vi "AlliGator Load IRFs & Fit Data (Map) HDF5 File v0.7.vi"(8 "Error In":errorcluster, 9 "File Type & Version only":bool, 11 "File Path":path) -> (0 "error out":errorcluster, 1 "Data Description":string, 2 "Decay Fit Options & Parameters":T1={"SYNC Period"=0.0, "Fit Options"={"Show Fit Residuals"=FALSE, "Fit Model"=enum."1-Exponential", "Residual Type"=enum."Standard", "Max Decay Percentile"=0.0, "Min Decay Percentile"=0.0, "Show Full Decay"=FALSE, "Weights"=enum."Unweighted", "Fitting Method"=enum."Least Square", "Compute Parameter Uncertainties"=FALSE, "Periodic Boundaries"=FALSE, "Model Calculation"=enum."Simulation", "Period"=0.0, "Termination Criteria"={"Max Iterations"=0, "Max Function Calls"=0, "Max Time"=0.0, "Function Tolerance"=0.0, "Parameter Tolerance"=0.0, "Gradient Tolerance"=0.0, "Min Lambda"=0.0, "Max Lambda"=0.0, "Initial Tick Count"=0}, "Offset Resolution"=0.0, "Use Local IRF"=FALSE, "Fitting Algorithm"=enum."Levenberg-Marquardt", "Show Confidence Interval "=TRUE, "Confidence Level"=95.0}, "Fit Parameter Constraints"=[], "MLE Baseline Offset"=0.0, "MLE Baseline Offset Type"=enum."Absolute"} {"Fit Options"."Confidence Level" min=0.0 max=100.0; "Fit Options"."Offset Resolution" min=0.0; "Fit Options"."Period" min=0.0; "Fit Options"."Min Decay Percentile" min=0.0 max=1.0; "Fit Options"."Max Decay Percentile" min=0.0 max=100.0; "Fit Parameter Constraints"."Max Value" format="%#.3g"; "Fit Parameter Constraints"."Min Value" format="%#.3g"}, 3 "IRFs & Fit Data Map v3":T13 {"Fit Options: Decay Preprocessing Parameters"."# Folds" min=1}, 4 "[Multiple Decays Fit Parameters SDV]":dbl[][](array[numeric]), 5 "File Version":string, 7 "File Type":string)   [LabVIEW 2021, in "AlliGator Decay Fit Parameter Map.lvlib"]
doc: "Loads Decay Fit Parameter Map and associated metadata."
uses:
  AlliGator Decay Fit Parameter Map.lvlib
  AlliGator IRFs & Fit Data v3.ctl
  Fits/IRF(X)PSED/Decay Fit Parameters & Derived Quantities List v2.ctl
  Decay Analysis/Decay Preprocessing/AlliGator Decay Preprocessing Parameters.ctl
  Graphs/XY Graph/XY Graph Plot Shift Parameters.ctl
  Graphs/XY Graph/XY Graph Plot Shift Method.ctl
  Fits/Decay Convolution/Decay Model.ctl
  Fits/Residual Type.ctl
  Fits/Non-linear Fitting Method v2.ctl
  Fits/Fit Calculation Method.ctl
  Fits/Non-linear Fitting Algorithm.ctl
  Decay Analysis/Decay Fit/AlliGator Decay Fit Parameter Constraints 2.ctl
  Fits/IRF(X)PSED/Decay Fit Parameters In List.ctl
  Fits/IRF(X)PSED/MLE Baseline Offset Type.ctl
  Fits/IRF(X)PSED/Decay Fit Options v1.ctl
  Fits/Non-linear Fitting Method v1.ctl
  AlliGator IRFs & Fit Data v1.ctl
  Decay Analysis/Decay Fit/AlliGator Decay Fit Options & Parameters v1.ctl
  AlliGator IRFs & Fit Data v2.ctl
  AlliGator Decay Fit Options & Parameters v2.ctl
  Fits/IRF(X)PSED/Decay Fit Options v2.ctl
  <vilib>/addons/h5labview2/base/lib_path.vi
  <vilib>/addons/h5labview2/base/H5Equery.vi
  <vilib>/addons/h5labview2/base/hid_t.ctl
  <vilib>/addons/h5labview2/dataset/H5Dread.llb/H5Dread.xnode
  <vilib>/addons/h5labview2/file/H5F.lvlib
  <vilib>/addons/h5labview2/group/H5G.lvlib
  Time/Time.lvlib
  Fits/Fits.lvlib
  Strings/Strings.lvlib
  Decay Analysis/Decay Fit/AlliGator Decay Fit.lvlib
  Fits/IRF(X)PSED/Fit Weights Type.ctl
  Graphs/XY Graph/XY Graph Add-Ons.lvlib
  Decay Analysis/Decay Preprocessing/AlliGator Decay Preprocessing.lvlib
  AlliGator Decay Fit Options & Parameters v3.ctl
  Fits/IRF(X)PSED/Decay Fit Options v3.ctl
  Fits/IRF(X)PSED/Fit Weights Type v2.ctl
  Fits/IRF(X)PSED/Decay Fit Options v4.ctl
  AlliGator Decay Fit Options & Parameters v4.ctl
panel:
  in  "Fit Parameter":T12(ring)
  out "elapsed (relative) seconds":dbl
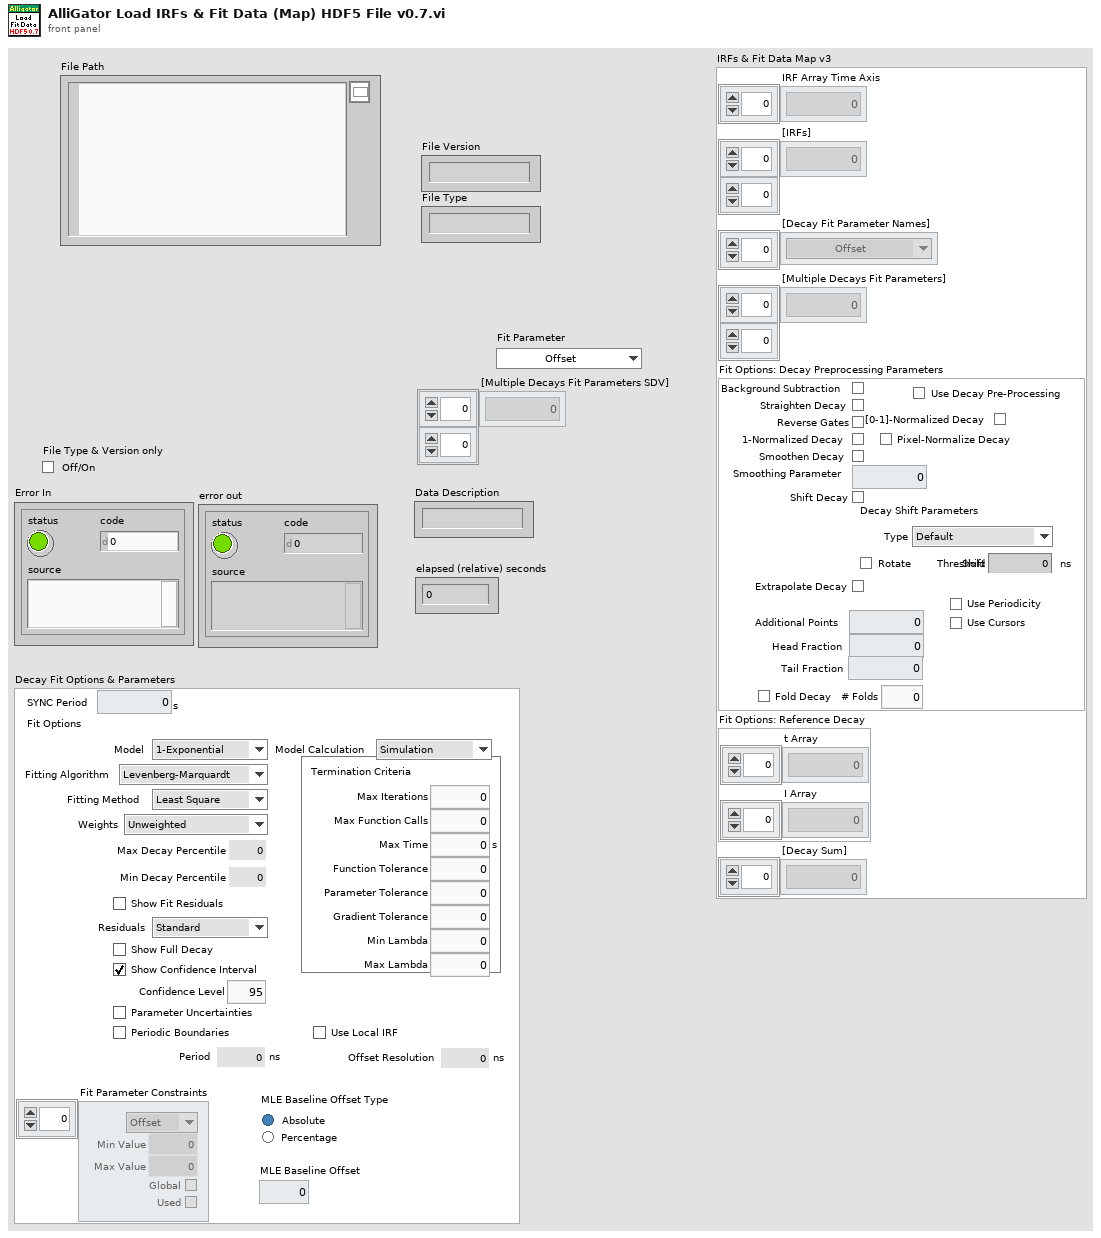
[diagram p1: front panel]
types:
  T1 = typedef "AlliGator Decay Fit Parameter Map.lvlib/AlliGator Decay Fit Options & Parameters v4.ctl" = cluster{"SYNC Period":dbl[unit], "Fit Options":T2, "Fit Parameter Constraints":T9[], "MLE Baseline Offset":dbl, "MLE Baseline Offset Type":T11}
  T2 = typedef "Fits.lvlib/Decay Fit Options v4.ctl" = cluster{"Show Fit Residuals":bool, "Fit Model":T3, "Residual Type":T4, "Max Decay Percentile":dbl, "Min Decay Percentile":dbl, "Show Full Decay":bool, "Weights":T5, "Fitting Method":T6, "Compute Parameter Uncertainties":bool, "Periodic Boundaries":bool, "Model Calculation":T7, "Period":dbl[unit], "Termination Criteria":cluster{"Max Iterations":i32, "Max Function Calls":i32, "Max Time":dbl[unit], "Function Tolerance":dbl, "Parameter Tolerance":dbl, "Gradient Tolerance":dbl, "Min Lambda":dbl, "Max Lambda":dbl, "Initial Tick Count":u32}, "Offset Resolution":dbl[unit], "Use Local IRF":bool, "Fitting Algorithm":T8, "Show Confidence Interval ":bool, "Confidence Level":dbl}
  T3 = typedef "Fits.lvlib/Decay Model.ctl" = enum16{"1-Exponential", "2-Exponentials"}
  T4 = typedef "Fits.lvlib/Residual Type.ctl" = enum16{"Standard", "Normalized", "Reduced"}
  T5 = typedef "Fits.lvlib/Fit Weights Type v2.ctl" = enum16{"Unweighted", "1/Variance (Neyman)", "1/Variance (Pearson)", "Best of All"}
  T6 = typedef "Fits.lvlib/Non-linear Fitting Method v2.ctl" = enum16{"Least Square", "Least Absolute Residual", "Bisquare", "MLE", "-", "Best of All"}
  T7 = typedef "Fits.lvlib/Fit Calculation Method.ctl" = enum16{"Simulation", "Convolution", "Integration"}
  T8 = typedef "Fits.lvlib/Non-linear Fitting Algorithm.ctl" = enum16{"Levenberg-Marquardt", "Trust-Region Dogleg"}
  T9 = typedef "AlliGator Decay Fit.lvlib/AlliGator Decay Fit Parameter Constraints 2.ctl" = cluster{"Fit Parameter":T10, "Min Value":dbl, "Max Value":dbl, "Global":bool, "Used":bool}
  T10 = typedef "Fits.lvlib/Decay Fit Parameters In List.ctl" = enum16{"Offset", "Baseline", "A_1", "tau_1", "A_2", "tau_2"}
  T11 = typedef "Fits.lvlib/MLE Baseline Offset Type.ctl" = enum32{"Absolute", "Percentage"}
  T12 = enum16{"Offset", "Baseline", "A_1", "tau_1", "A_2", "tau_2", "<tau>_1", "f1_1", "f2_1", "<tau>_2", "f1_2", "f2_2", "-", "R^2", "Chi^2"}
  T13 = typedef "AlliGator Decay Fit Parameter Map.lvlib/AlliGator IRFs & Fit Data v3.ctl" = cluster{"IRF Array Time Axis":dbl[], "[IRFs]":dbl[][], "[Decay Fit Parameter Names]":T14[], "[Multiple Decays Fit Parameters]":dbl[][], "Fit Options: Decay Preprocessing Parameters":T15, "Fit Options: Reference Decay":cluster{"t Array":dbl[], "I Array":dbl[]}, "[Decay Sum]":dbl[]}
  T14 = typedef "Fits.lvlib/Decay Fit Parameters & Derived Quantities List v2.ctl" = enum16{"Offset", "Baseline", "A_1", "tau_1", "A_2", "tau_2", "<tau>_a", "f1_a", "f2_a", "<tau>_i", "f1_i", "f2_i", "-", "R^2", "Chi^2"}
  T15 = typedef "AlliGator Decay Preprocessing.lvlib/AlliGator Decay Preprocessing Parameters.ctl" = cluster{"Background Subtraction":bool, "Straighten Decay":bool, "Reverse Gates":bool, "1-Normalized Decay":bool, "Smoothen Decay":bool, "Smoothing Parameter":dbl, "Shift Decay":bool, "Decay Shift Parameters":T16, "Extrapolate Decay":bool, "Additional Points":u32, "Head Fraction":dbl, "Pixel-Normalize Decay":bool, "Use Periodicity":bool, "Use Cursors":bool, "Tail Fraction":dbl, "Use Decay Pre-Processing":bool, "Fold Decay":bool, "# Folds":u32, "[0-1]-Normalized Decay":bool}
  T16 = typedef "XY Graph Add-Ons.lvlib/XY Graph Plot Shift Parameters.ctl" = cluster{"Type":T17, "Shift":dbl[unit], "Threshold":dbl, "Rotate":bool}
  T17 = typedef "XY Graph Add-Ons.lvlib/XY Graph Plot Shift Method.ctl" = enum16{"Default", "CFD", "Threshold", "Cross-Correlation"}
  T18 = typedef "AlliGator Decay Fit.lvlib/AlliGator Decay Fit Options & Parameters v1.ctl" = cluster{"SYNC Period":dbl[unit], "Fit Options":T19, "Fit Parameter Constraints":T9[]}
  T19 = typedef "Fits.lvlib/Decay Fit Options v1.ctl" = cluster{"Show Fit Residuals":bool, "Fit Model":T3, "Residual Type":T4, "Max Decay Percentile":dbl, "Min Decay Percentile":dbl, "Show Full Decay":bool, "Weights":T20, "Fitting Method":T21, "Compute Parameter Uncertainties":bool, "Periodic Boundaries":bool, "Model Calculation":T7, "Period":dbl[unit], "Termination Criteria":cluster{"Max Iterations":i32, "Max Function Calls":i32, "Max Time":dbl[unit], "Function Tolerance":dbl, "Parameter Tolerance":dbl, "Gradient Tolerance":dbl, "Min Lambda":dbl, "Max Lambda":dbl, "Initial Tick Count":u32}, "Offset Resolution":dbl[unit], "Use Local IRF":bool, "Fitting Algorithm":T8}
  T20 = typedef "Fits.lvlib/Fit Weights Type.ctl" = enum16{"Unweighted", "1/Variance", "Best of All"}
  T21 = typedef "Fits.lvlib/Non-linear Fitting Method v1.ctl" = enum16{"Least Square", "Least Absolute Residual", "Bisquare", "-", "Best of All"}
  T22 = typedef "AlliGator Decay Fit Parameter Map.lvlib/AlliGator IRFs & Fit Data v1.ctl" = cluster{"IRF Array Time Axis":dbl[], "[IRF]":dbl[][], "[Decay Fit Parameter Name]":T14[], "[Multiple Decays Fit Parameters]":dbl[][]}
  T23 = typedef "AlliGator Decay Fit Parameter Map.lvlib/AlliGator IRFs & Fit Data v2.ctl" = cluster{"IRF Array Time Axis":dbl[], "[IRFs]":dbl[][], "[Decay Fit Parameter Names]":T14[], "[Multiple Decays Fit Parameters]":dbl[][], "Fit Options: Decay Preprocessing Parameters":T15, "Fit Options: Reference Decay":cluster{"t Array":dbl[], "I Array":dbl[]}}
  T24 = typedef "AlliGator Decay Fit Parameter Map.lvlib/AlliGator Decay Fit Options & Parameters v2.ctl" = cluster{"SYNC Period":dbl[unit], "Fit Options":T25, "Fit Parameter Constraints":T9[], "MLE Baseline Offset":dbl, "MLE Baseline Offset Type":T11}
  T25 = typedef "Fits.lvlib/Decay Fit Options v2.ctl" = cluster{"Show Fit Residuals":bool, "Fit Model":T3, "Residual Type":T4, "Max Decay Percentile":dbl, "Min Decay Percentile":dbl, "Show Full Decay":bool, "Weights":T20, "Fitting Method":T6, "Compute Parameter Uncertainties":bool, "Periodic Boundaries":bool, "Model Calculation":T7, "Period":dbl[unit], "Termination Criteria":cluster{"Max Iterations":i32, "Max Function Calls":i32, "Max Time":dbl[unit], "Function Tolerance":dbl, "Parameter Tolerance":dbl, "Gradient Tolerance":dbl, "Min Lambda":dbl, "Max Lambda":dbl, "Initial Tick Count":u32}, "Offset Resolution":dbl[unit], "Use Local IRF":bool, "Fitting Algorithm":T8}
  T26 = typedef "AlliGator Decay Fit Parameter Map.lvlib/AlliGator Decay Fit Options & Parameters v3.ctl" = cluster{"SYNC Period":dbl[unit], "Fit Options":T27, "Fit Parameter Constraints":T9[], "MLE Baseline Offset":dbl, "MLE Baseline Offset Type":T11}
  T27 = typedef "Fits.lvlib/Decay Fit Options v3.ctl" = cluster{"Show Fit Residuals":bool, "Fit Model":T3, "Residual Type":T4, "Max Decay Percentile":dbl, "Min Decay Percentile":dbl, "Show Full Decay":bool, "Weights":T20, "Fitting Method":T6, "Compute Parameter Uncertainties":bool, "Periodic Boundaries":bool, "Model Calculation":T7, "Period":dbl[unit], "Termination Criteria":cluster{"Max Iterations":i32, "Max Function Calls":i32, "Max Time":dbl[unit], "Function Tolerance":dbl, "Parameter Tolerance":dbl, "Gradient Tolerance":dbl, "Min Lambda":dbl, "Max Lambda":dbl, "Initial Tick Count":u32}, "Offset Resolution":dbl[unit], "Use Local IRF":bool, "Fitting Algorithm":T8, "Show Confidence Interval ":bool, "Confidence Level":dbl}
  T28 = typedef "hid_t.ctl" = i64
  T29 = cluster{"Laser Period":dbl[unit], "Fit Options":T19, "Fit Parameter Constraints":T9[]}
  T30 = cluster{"IRF Array Time Axis":dbl[], "[IRF]":dbl[][], "[Decay Fit Parameter Name]":T14[], "[Multiple Decays Fit Parameters]":dbl[][]}
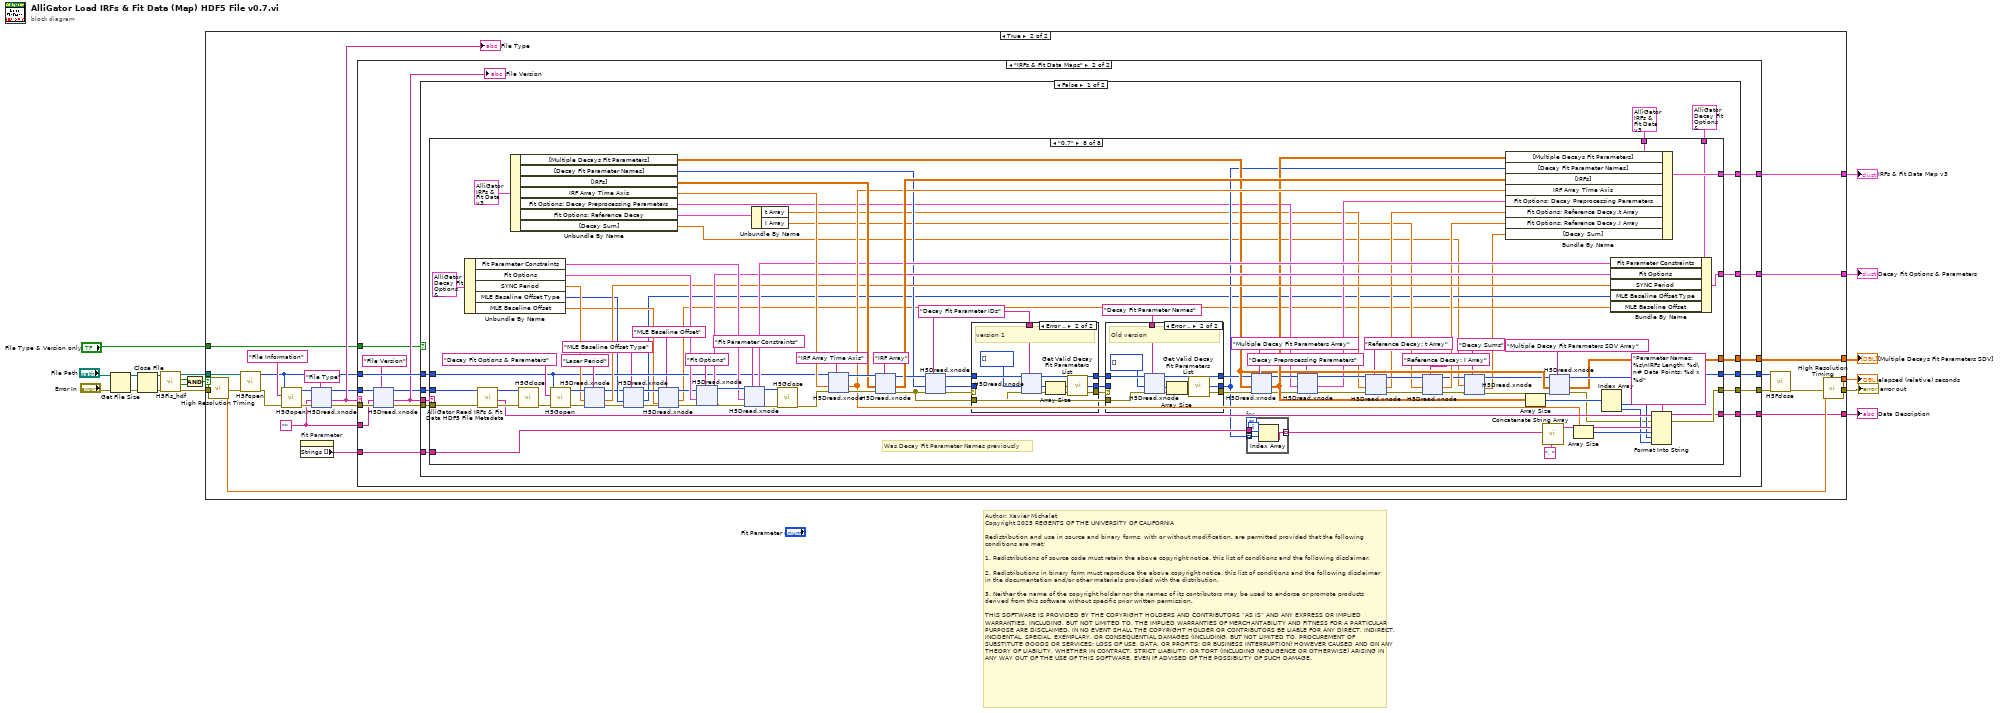
[diagram p0: block diagram]
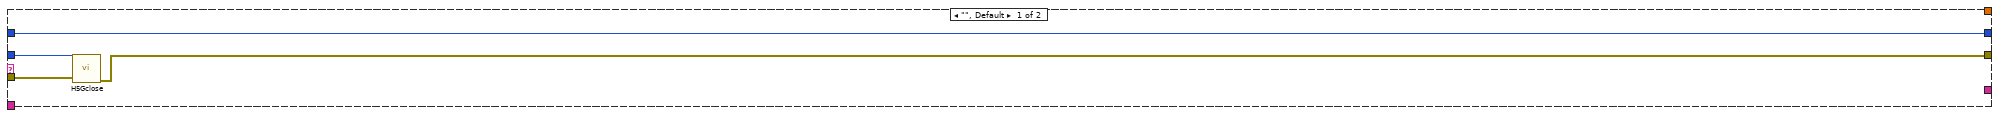
[diagram p3: hidden frame]
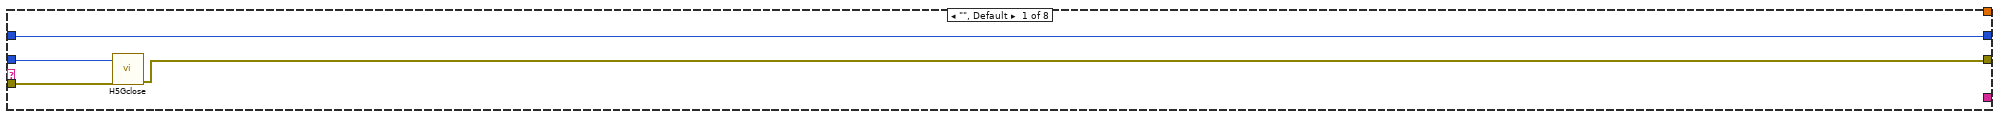
[diagram p4: hidden frame]
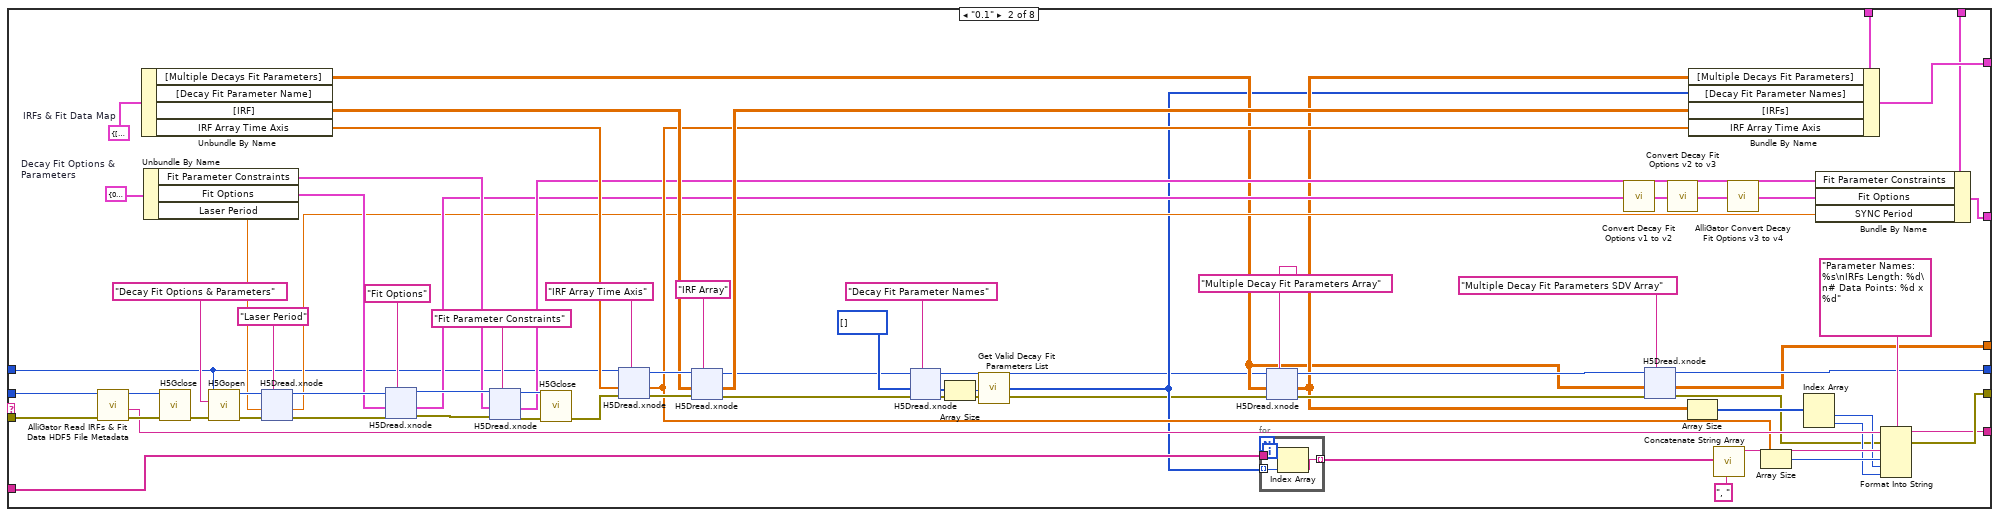
[diagram p5: hidden frame]
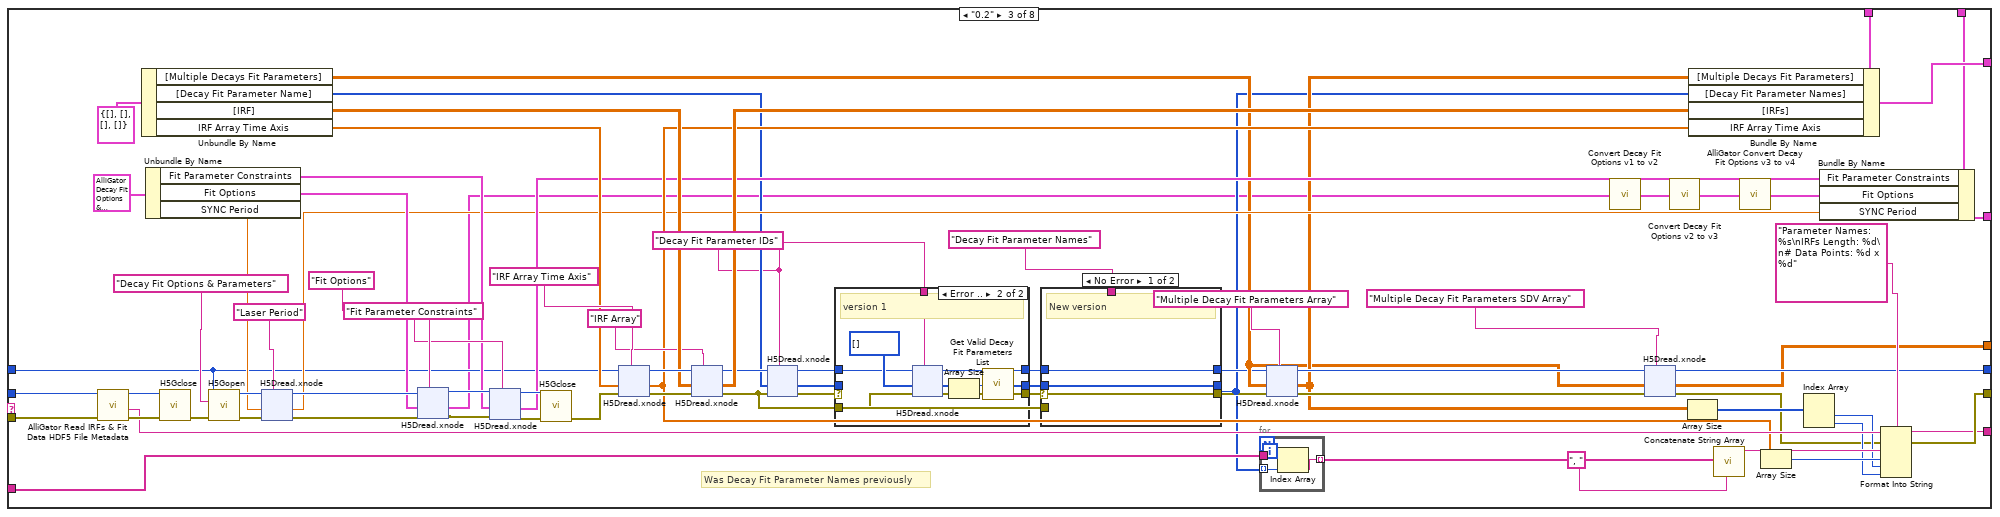
[diagram p6: hidden frame]
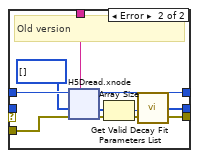
[diagram p8: hidden frame]
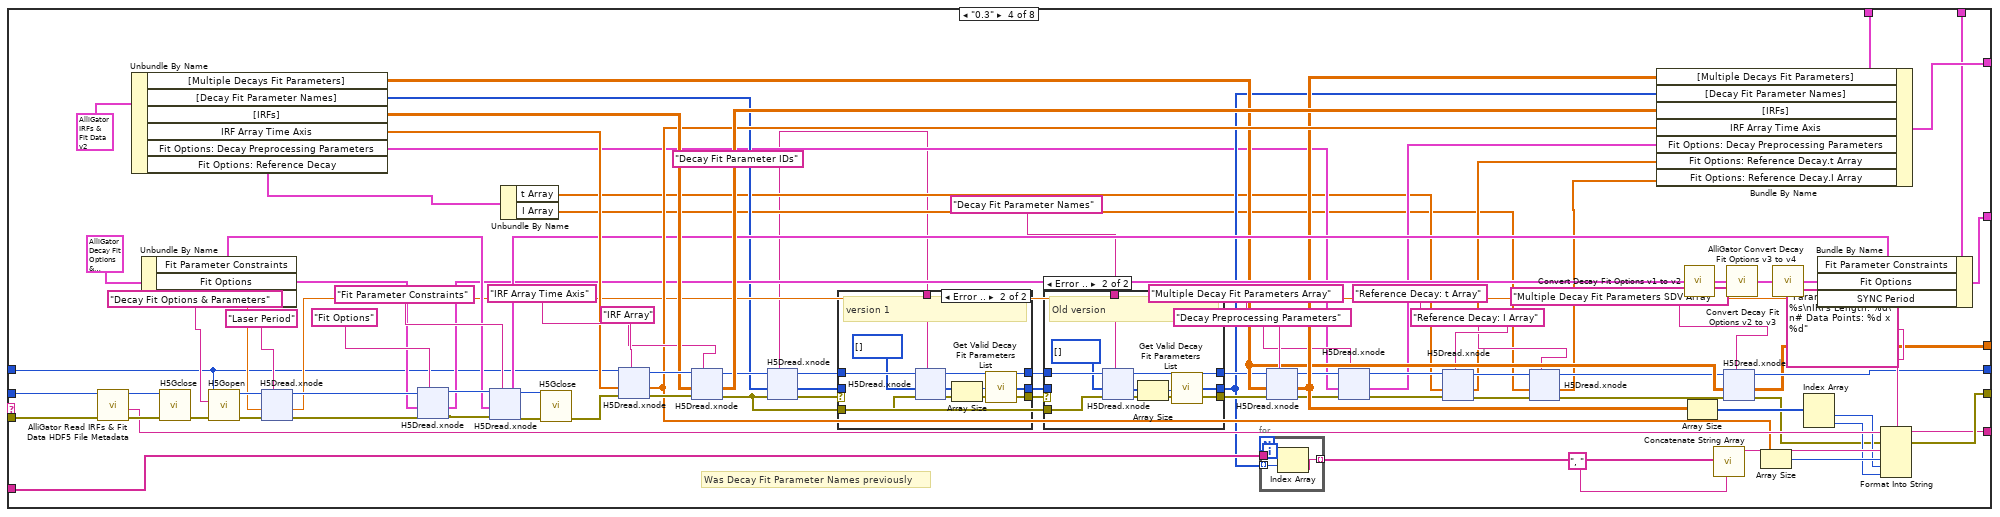
[diagram p9: hidden frame]
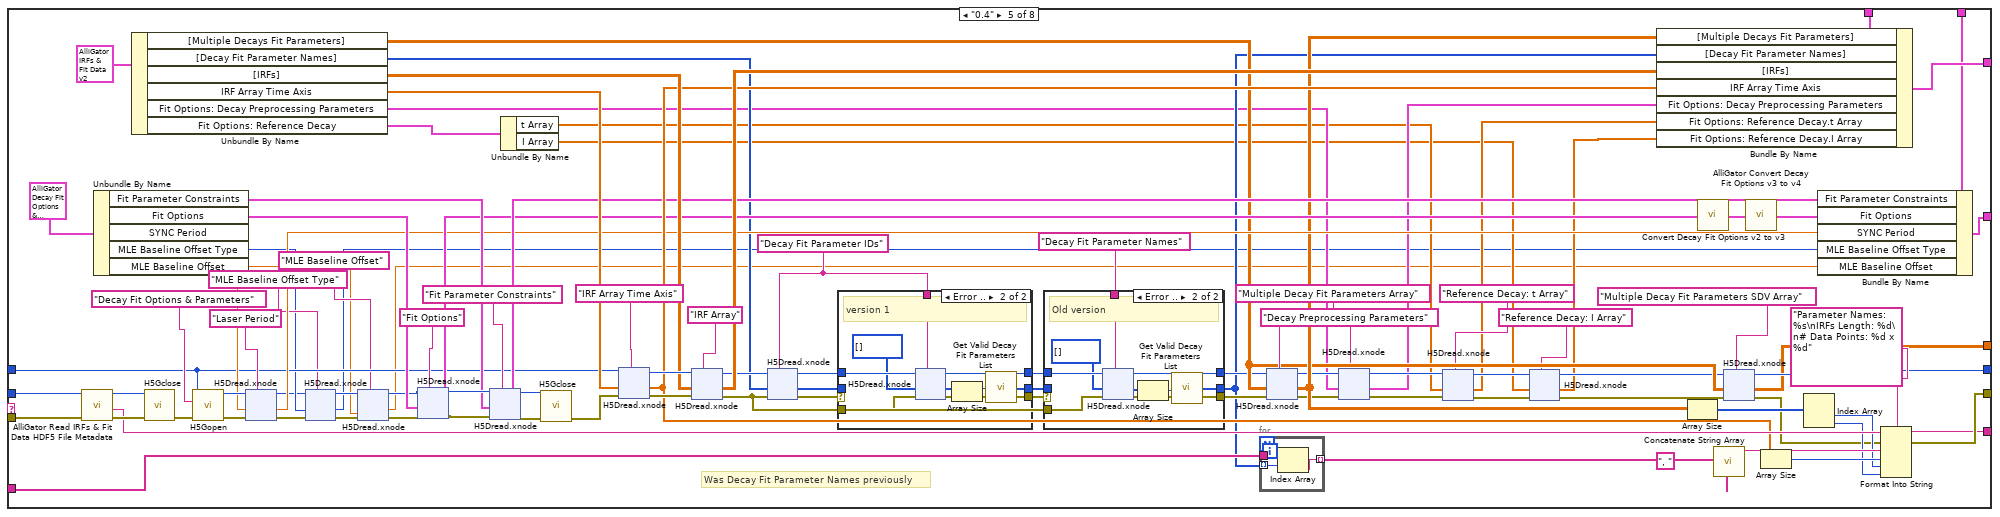
[diagram p12: hidden frame]
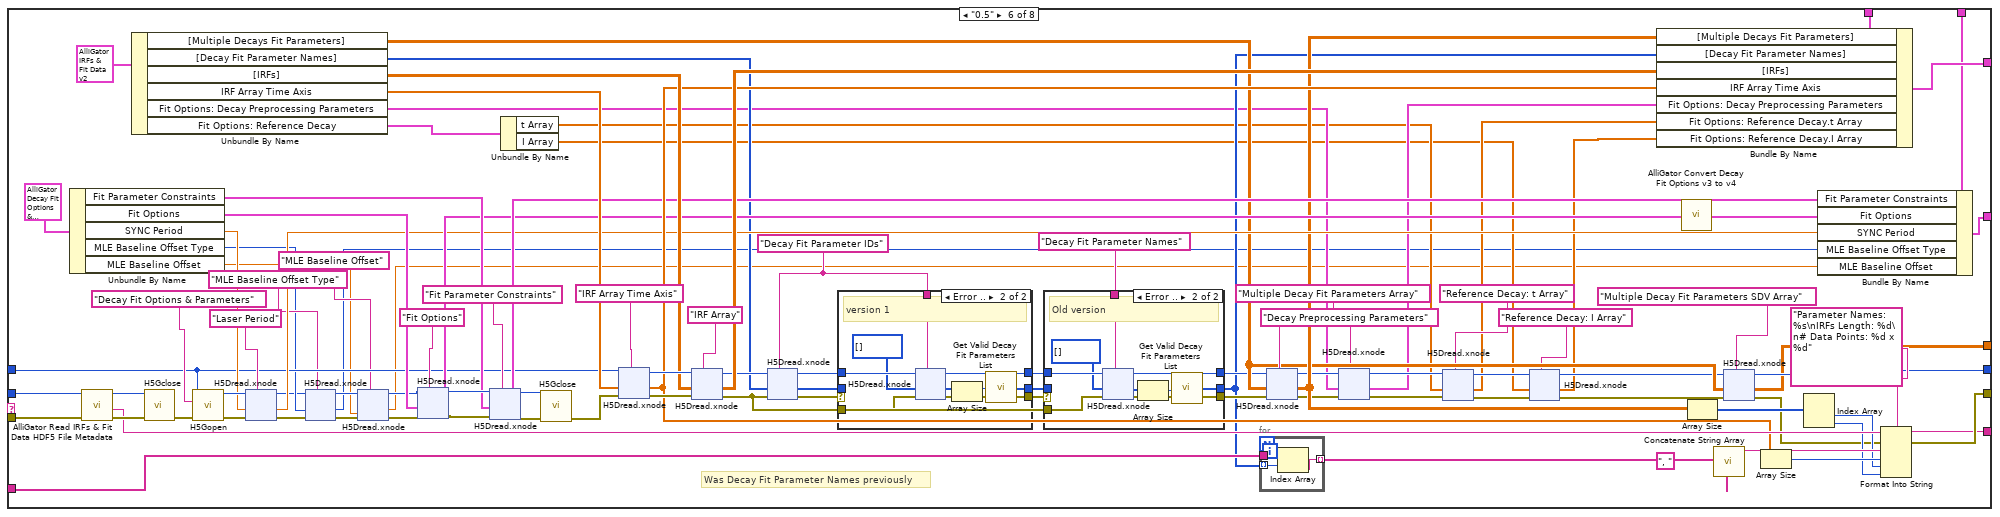
[diagram p15: hidden frame]
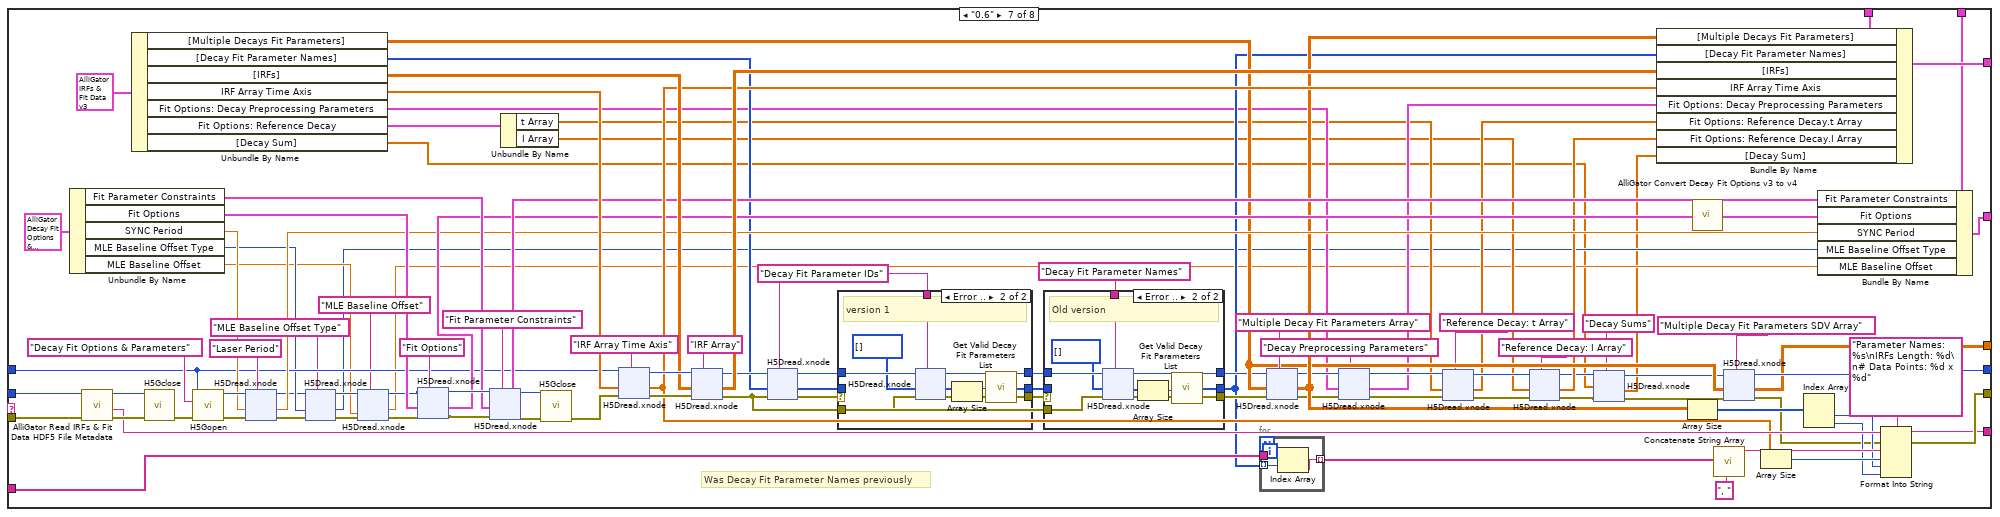
[diagram p18: hidden frame]
diagram:
  # "Author: Xavier Michalet\nCopyright 2025 REGENTS OF THE UNIVERSITY OF CALIFORNIA\n\nRedistribution and use in source and binary forms, with or without modification, are permitted provided that the following conditions are met:\n\n1. Redistributions of source code must retain the above copyright notice, this list of conditions and the following disclaimer.\n\n2. Redistributions in binary form must reproduce the above copyright notice, this list of conditions and the following disclaimer in the documentation and/or other materials provided with the distribution.\n\n3. Neither the name of the copyright holder nor the names of its contributors may be used to endorse or promote products derived from this software without specific prior written permission.\n\nTHIS SOFTWARE IS PROVIDED BY THE COPYRIGHT HOLDERS AND CONTRIBUTORS “AS IS” AND ANY EXPRESS OR IMPLIED WARRANTIES, INCLUDING, BUT NOT LIMITED TO, THE IMPLIED WARRANTIES OF MERCHANTABILITY AND FITNESS FOR A PARTICULAR PURPOSE ARE DISCLAIMED. IN NO EVENT SHALL THE COPYRIGHT HOLDER OR CONTRIBUTORS BE LIABLE FOR ANY DIRECT, INDIRECT, INCIDENTAL, SPECIAL, EXEMPLARY, OR CONSEQUENTIAL DAMAGES (INCLUDING, BUT NOT LIMITED TO, PROCUREMENT OF SUBSTITUTE GOODS OR SERVICES; LOSS OF USE, DATA, OR PROFITS; OR BUSINESS INTERRUPTION) HOWEVER CAUSED AND ON ANY THEORY OF LIABILITY, WHETHER IN CONTRACT, STRICT LIABILITY, OR TORT (INCLUDING NEGLIGENCE OR OTHERWISE) ARISING IN ANY WAY OUT OF THE USE OF THIS SOFTWARE, EVEN IF ADVISED OF THE POSSIBILITY OF SUCH DAMAGE."
  n1 = Get File Size(file="File Path", error in="Error In") -> (refnum out=w9:refnum<file>, 0:w10:errorcluster)  [unwired: 1 out]
  n2 = Close File(refnum=w9, error in=w10) -> (path=w8:path, error out=w7:errorcluster)
  n3 = call <vilib>:"H5Fis_hdf.vi"("error in (no error)"=w7, "path in"=w8) -> ("error out"=w14:errorcluster, "valid?"=w17:bool, "exists?"=w18:bool, "path out"=w15:path)  [unwired: 6 in]
  n4 = And(x=w18, y=w17) -> (x .and. y?=w16:bool)
  n5 = case shown="True" w16 {
    tunnel: w15 -> [_ w27]
    tunnel: w14 -> [w19 w44]
    tunnel: [w19 w39] -> w13
    tunnel: [_ w37] -> w6
    tunnel: [_ w26] -> w5
    tunnel: [_ w24] -> w4
    tunnel: [_ w22] -> w3
    tunnel: "File Type & Version only" -> [_ w21]
    tunnel: [_ w20] -> w1
    frame False {
    }
    frame True {
      w28 = ""
      n6 = call "High Resolution Timing.vi"("Error In"=w44) -> ("elapsed (relative) seconds"=w38:dbl, "Error Out"=w40:errorcluster)  [unwired: 16 in, 1 out]
      n7 = call <vilib>:"H5Fopen.vi"("error in (no error)"=w40, "path"=w27) -> ("error out"=w36:errorcluster, "ref out"=w31:T28)  [unwired: 8 in]
      n8 = call <vilib>:"H5Gopen.vi"("error in (no error)"=w36, "name"="File Information" ("dataset name (this)"), "ref in"=w31) -> ("error out"=w34:errorcluster, "group out"=w33:T28)  [unwired: 7 in]
      n9 = property on="Fit Parameter" class="Enum (strict)"() -> ("Strings []"=w23:string[])  [unwired: 2 in, 2 out]
      n10 = xnode "H5Dread.xnode"("dataset name (this)"="File Type", "error in (no error)"=w34, "default"=w28, "ref in"=w33) -> ("error out"=w30:errorcluster, "data"=w43:string, "ref out"=w29:T28)  [unwired: 2 in, 1 out]
      "File Type" <- w43
      n11 = case shown="\"IRFs & Fit Data Maps\"" w43 {
        tunnel: [w48 w64] -> w42
        tunnel: [w45 w57] -> w41
        tunnel: w31 -> [w48 w63]
        tunnel: w30 -> [w47 w61]
        tunnel: w28 -> [_ w60]
        tunnel: w29 -> [w46 w59]
        tunnel: [_ w56] -> w26
        tunnel: [_ w53] -> w24
        tunnel: w23 -> [_ w52]
        tunnel: [_ w51] -> w22
        tunnel: w21 -> [_ w50]
        tunnel: [_ w49] -> w20
        frame "", Default {
          n12 = call <vilib>:"H5Gclose.vi"("error in (no error)"=w47, "group in"=w46) -> ("error out"=w45:errorcluster)  [unwired: 9 in]
        }
        frame "IRFs & Fit Data Maps" {
          n13 = xnode "H5Dread.xnode"("dataset name (this)"="File Version", "error in (no error)"=w61, "default"=w60, "ref in"=w59) -> ("error out"=w55:errorcluster, "data"=w58:string, "ref out"=w54:T28)  [unwired: 2 in, 1 out]
          "File Version" <- w58
          n14 = case shown="False" w50 {
            tunnel: [w77 w2295] -> w64
            tunnel: w63 -> [w76 w2295]
            tunnel: w58 -> [w75 _]
            tunnel: [w74 w2294] -> w57
            tunnel: [w73 _] -> w56
            tunnel: w55 -> [w72 w2297]
            tunnel: w54 -> [w71 w2296]
            tunnel: [w70 _] -> w53
            tunnel: w52 -> [w69 _]
            tunnel: [w68 _] -> w51
            tunnel: [w67 _] -> w49
            frame False {
              n15 = case shown="\"0.7\"" w75 {
                tunnel: w76 -> [w81 w104 w304 w573 w898 w1250 w1607 w1978]
                tunnel: [w81 w100 w300 w571 w896 w1248 w1605 w1976] -> w77
                tunnel: [w78 w139 w338 w608 w931 w1283 w1640 w2011] -> w74
                tunnel: [_ w144 w343 w613 w936 w1288 w1645 w2016] -> w73
                tunnel: w72 -> [w80 w142 w341 w611 w934 w1286 w1643 w2014]
                tunnel: w71 -> [w79 w143 w342 w612 w935 w1287 w1644 w2015]
                tunnel: [_ w138 w337 w607 w930 w1282 w1639 w2010] -> w70
                tunnel: w69 -> [_ w135 w334 w604 w927 w1279 w1636 w2007]
                tunnel: [_ w105 w305 w574 w899 w1251 w1608 w1979] -> w68
                tunnel: [_ w96 w296 w567 w892 w1244 w1601 w1972] -> w67
                tunnel: T13 {"IRF Array Time Axis"=[], "[IRFs]"=[], "[Decay Fit Parameter Names]"=[], "[Multiple Decays Fit Parameters]"=[], "Fit Options: Decay Preprocessing Parameters"={"Background Subtraction"=FALSE, "Straighten Decay"=FALSE, "Reverse Gates"=FALSE, "1-Normalized Decay"=FALSE, "Smoothen Decay"=FALSE, "Smoothing Parameter"=0.0, "Shift Decay"=FALSE, "Decay Shift Parameters"={"Type"=enum."Default", "Shift"=0.0, "Threshold"=0.0, "Rotate"=FALSE}, "Extrapolate Decay"=FALSE, "Additional Points"=0, "Head Fraction"=0.0, "Pixel-Normalize Decay"=FALSE, "Use Periodicity"=FALSE, "Use Cursors"=FALSE, "Tail Fraction"=0.0, "Use Decay Pre-Processing"=FALSE, "Fold Decay"=FALSE, "# Folds"=0, "[0-1]-Normalized Decay"=FALSE}, "Fit Options: Reference Decay"={"t Array"=[], "I Array"=[]}, "[Decay Sum]"=[]} ("IRFs & Fit Data Map") -> [_ w95 w294 w561 w886 w1238 w1595 w1966]
                tunnel: T1 {"SYNC Period"=0.0, "Fit Options"={"Show Fit Residuals"=FALSE, "Fit Model"=enum."1-Exponential", "Residual Type"=enum."Standard", "Max Decay Percentile"=0.0, "Min Decay Percentile"=0.0, "Show Full Decay"=FALSE, "Weights"=enum."Unweighted", "Fitting Method"=enum."Least Square", "Compute Parameter Uncertainties"=FALSE, "Periodic Boundaries"=FALSE, "Model Calculation"=enum."Simulation", "Period"=0.0, "Termination Criteria"={"Max Iterations"=0, "Max Function Calls"=0, "Max Time"=0.0, "Function Tolerance"=0.0, "Parameter Tolerance"=0.0, "Gradient Tolerance"=0.0, "Min Lambda"=0.0, "Max Lambda"=0.0, "Initial Tick Count"=0}, "Offset Resolution"=0.0, "Use Local IRF"=FALSE, "Fitting Algorithm"=enum."Levenberg-Marquardt", "Show Confidence Interval "=TRUE, "Confidence Level"=95.0}, "Fit Parameter Constraints"=[], "MLE Baseline Offset"=0.0, "MLE Baseline Offset Type"=enum."Absolute"} ("Decay Fit Options & Parameters") -> [_ w85 w281 w534 w859 w1211 w1570 w1941]
                frame "", Default {
                  n16 = call <vilib>:"H5Gclose.vi"("error in (no error)"=w80, "group in"=w79) -> ("error out"=w78:errorcluster)  [unwired: 9 in]
                }
                frame "0.1" {
                  w109 = T29 {"Laser Period"=0.0, "Fit Options"={"Show Fit Residuals"=FALSE, "Fit Model"=enum."1-Exponential", "Residual Type"=enum."Standard", "Max Decay Percentile"=0.0, "Min Decay Percentile"=0.0, "Show Full Decay"=FALSE, "Weights"=enum."Unweighted", "Fitting Method"=enum."Least Square", "Compute Parameter Uncertainties"=FALSE, "Periodic Boundaries"=FALSE, "Model Calculation"=enum."Simulation", "Period"=0.0, "Termination Criteria"={"Max Iterations"=0, "Max Function Calls"=0, "Max Time"=0.0, "Function Tolerance"=0.0, "Parameter Tolerance"=0.0, "Gradient Tolerance"=0.0, "Min Lambda"=0.0, "Max Lambda"=0.0, "Initial Tick Count"=0}, "Offset Resolution"=0.0, "Use Local IRF"=FALSE, "Fitting Algorithm"=enum."Levenberg-Marquardt"}, "Fit Parameter Constraints"=[]}  # Decay Fit Options & Parameters
                  w149 = T30 {"IRF Array Time Axis"=[], "[IRF]"=[], "[Decay Fit Parameter Name]"=[], "[Multiple Decays Fit Parameters]"=[]}  # IRFs & Fit Data Map
                  n17 = call "AlliGator Read IRFs & Fit Data HDF5 File Metadata.vi"("error in (no error)"=w142, "ref in"=w143) -> ("error out"=w140:errorcluster, "File Metadata"=w137:string, "ref out"=w141:T28)  [unwired: 7 in]
                  n18 = Unbundle By Name(w149) -> ("[Multiple Decays Fit Parameters]"=w97:dbl[][], "[IRF]"=w148:dbl[][], "IRF Array Time Axis"=w150:dbl[])  [unwired: 1 out]
                  n19 = Unbundle By Name(w109) -> ("Fit Parameter Constraints"=w110:T9[], "Fit Options"=w111:T19, "Laser Period"=w112:dbl[unit])
                  n20 = call <vilib>:"H5Gclose.vi"("error in (no error)"=w140, "group in"=w141) -> ("error out"=w115:errorcluster)  [unwired: 9 in]
                  n21 = call <vilib>:"H5Gopen.vi"("error in (no error)"=w115, "name"="Decay Fit Options & Parameters" ("dataset name"), "ref in"=w104) -> ("error out"=w126:errorcluster, "group out"=w125:T28)  [unwired: 7 in]
                  n22 = xnode "H5Dread.xnode"("dataset name (this)"="Laser Period" ("dataset name"), "error in (no error)"=w126, "default"=w112, "ref in"=w125) -> ("error out"=w124:errorcluster, "data"=w106:dbl[unit], "ref out"=w121:T28)  [unwired: 2 in, 1 out]
                  n23 = xnode "H5Dread.xnode"("dataset name (this)"="Fit Options" ("dataset name"), "error in (no error)"=w124, "default"=w111, "ref in"=w121) -> ("error out"=w123:errorcluster, "data"=w107:T19, "ref out"=w120:i64)  [unwired: 2 in, 1 out]
                  n24 = xnode "H5Dread.xnode"("dataset name (this)"="Fit Parameter Constraints" ("dataset name"), "error in (no error)"=w123, "default"=w110, "ref in"=w120) -> ("error out"=w122:errorcluster, "data"=w108:T9[], "ref out"=w119:i64)  [unwired: 2 in, 1 out]
                  n25 = call <vilib>:"H5Gclose.vi"("error in (no error)"=w122, "group in"=w119) -> ("error out"=w114:errorcluster)  [unwired: 9 in]
                  n26 = xnode "H5Dread.xnode"("dataset name (this)"="IRF Array Time Axis" ("dataset name"), "error in (no error)"=w114, "default"=w150, "ref in"=w104) -> ("error out"=w153:errorcluster, "data"=w130:dbl[], "ref out"=w152:T28)  [unwired: 2 in, 1 out]
                  n27 = xnode "H5Dread.xnode"("dataset name (this)"="IRF Array" ("dataset name"), "error in (no error)"=w153, "default"=w148, "ref in"=w152) -> ("error out"=w93:errorcluster, "data"=w146:dbl[][], "ref out"=w88:T28)  [unwired: 2 in, 1 out]
                  n28 = xnode "H5Dread.xnode"("dataset name (this)"="Decay Fit Parameter Names" ("name"), "error in (no error)"=w93, "default"=u16[] [], "ref in"=w88) -> ("error out"=w86:errorcluster, "data"=w91:u16[], "ref out"=w87:i64)  [unwired: 2 in, 1 out]
                  n29 = Array Size(array=w91) -> (size(s)=w90:i32)
                  n30 = call "Get Valid Decay Fit Parameters List.vi"("Parameter ID Array Size"=w90) -> ("Parameter Name Array"=w89:T14[])
                  n31 = for {
                    tunnel: w135 -> [w231]
                    tunnel: [w230] -> w134 mode=indexing
                    tunnel: w89 -> [w229] mode=indexing
                    n32 = Index Array(array=w231, index=w229) -> (element=w230:string)
                  }
                  n33 = xnode "H5Dread.xnode"("dataset name (this)"="Multiple Decay Fit Parameters Array" ("name"), "error in (no error)"=w86, "default"=w97, "ref in"=w87) -> ("error out"=w103:errorcluster, "data"=w98:dbl[][], "ref out"=w101:T28)  [unwired: 2 in, 1 out]
                  n34 = call "Convert Decay Fit Options v1 to v2.vi"("Decay Fit Options v1"=w107) -> ("Decay Fit Options v2"=w84:T25)
                  n35 = xnode "H5Dread.xnode"("dataset name (this)"="Multiple Decay Fit Parameters SDV Array" ("name"), "error in (no error)"=w103, "default"=w97, "ref in"=w101) -> ("error out"=w102:errorcluster, "data"=w96:dbl[][], "ref out"=w100:T28)  [unwired: 2 in, 1 out]
                  n36 = call "Convert Decay Fit Options v2 to v3.vi"("Decay Fit Options v2"=w84) -> ("Decay Fit Options v3"=w83:T27)
                  n37 = Array Size(array=w98) -> (size(s)=w129:i32[])
                  n38 = Bundle By Name(cluster=w95, "[Multiple Decays Fit Parameters]"=w98, "[Decay Fit Parameter Names]"=w89, "[IRFs]"=w146, "IRF Array Time Axis"=w130) -> (w144:T13)
                  n39 = call "Concatenate String Array.vi"("Separator (TAB)"=", ", "String Array"=w134) -> ("Formatted String"=w132:string)  [unwired: 9 in]
                  n40 = call "AlliGator Convert Decay Fit Options v3 to v4.vi"("Decay Fit Options (v3)"=w83) -> ("Decay Fit Options (v4)"=w82:T2)
                  n41 = Array Size(array=w130) -> (size(s)=w131:i32)
                  n42 = Index Array(array=w129) -> (element #1=w128:i32, element #2=w127:i32)  [unwired: 2 in]
                  n43 = Bundle By Name(cluster=w85, "Fit Parameter Constraints"=w108, "Fit Options"=w82, "SYNC Period"=w106) -> (w105:T1)
                  n44 = Format Into String(format string="Parameter Names: %s\nIRFs Length: %d\n# Data Points: %d x %d", initial string=w137, error in=w102, w132, w131, w128, w127) -> (resulting string=w138:string, error out=w139:errorcluster)
                }
                frame "0.2" {
                  w289 = "Decay Fit Parameter IDs" ("name")
                  # "Was Decay Fit Parameter Names previously"
                  n45 = call "AlliGator Read IRFs & Fit Data HDF5 File Metadata.vi"("error in (no error)"=w341, "ref in"=w342) -> ("error out"=w339:errorcluster, "File Metadata"=w336:string, "ref out"=w340:T28)  [unwired: 7 in]
                  n46 = Unbundle By Name(T22 {"IRF Array Time Axis"=[], "[IRF]"=[], "[Decay Fit Parameter Name]"=[], "[Multiple Decays Fit Parameters]"=[]} ("IRFs & Fit Data Map")) -> ("[Multiple Decays Fit Parameters]"=w297:dbl[][], "[Decay Fit Parameter Name]"=w295:T14[], "[IRF]"=w348:dbl[][], "IRF Array Time Axis"=w350:dbl[])
                  n47 = Unbundle By Name(T18 {"SYNC Period"=0.0, "Fit Options"={"Show Fit Residuals"=FALSE, "Fit Model"=enum."1-Exponential", "Residual Type"=enum."Standard", "Max Decay Percentile"=0.0, "Min Decay Percentile"=0.0, "Show Full Decay"=FALSE, "Weights"=enum."Unweighted", "Fitting Method"=enum."Least Square", "Compute Parameter Uncertainties"=FALSE, "Periodic Boundaries"=FALSE, "Model Calculation"=enum."Simulation", "Period"=0.0, "Termination Criteria"={"Max Iterations"=0, "Max Function Calls"=0, "Max Time"=0.0, "Function Tolerance"=0.0, "Parameter Tolerance"=0.0, "Gradient Tolerance"=0.0, "Min Lambda"=0.0, "Max Lambda"=0.0, "Initial Tick Count"=0}, "Offset Resolution"=0.0, "Use Local IRF"=FALSE, "Fitting Algorithm"=enum."Levenberg-Marquardt"}, "Fit Parameter Constraints"=[]} ("Decay Fit Options & Parameters")) -> ("Fit Parameter Constraints"=w309:T9[], "Fit Options"=w310:T19, "SYNC Period"=w311:dbl[unit])
                  n48 = call <vilib>:"H5Gclose.vi"("error in (no error)"=w339, "group in"=w340) -> ("error out"=w314:errorcluster)  [unwired: 9 in]
                  n49 = call <vilib>:"H5Gopen.vi"("error in (no error)"=w314, "name"="Decay Fit Options & Parameters" ("dataset name"), "ref in"=w304) -> ("error out"=w325:errorcluster, "group out"=w324:T28)  [unwired: 7 in]
                  n50 = xnode "H5Dread.xnode"("dataset name (this)"="Laser Period" ("dataset name"), "error in (no error)"=w325, "default"=w311, "ref in"=w324) -> ("error out"=w323:errorcluster, "data"=w306:dbl[unit], "ref out"=w320:T28)  [unwired: 2 in, 1 out]
                  n51 = xnode "H5Dread.xnode"("dataset name (this)"="Fit Options" ("dataset name"), "error in (no error)"=w323, "default"=w310, "ref in"=w320) -> ("error out"=w322:errorcluster, "data"=w280:T19, "ref out"=w319:T28)  [unwired: 2 in, 1 out]
                  n52 = xnode "H5Dread.xnode"("dataset name (this)"="Fit Parameter Constraints" ("dataset name"), "error in (no error)"=w322, "default"=w309, "ref in"=w319) -> ("error out"=w321:errorcluster, "data"=w307:T9[], "ref out"=w318:T28)  [unwired: 2 in, 1 out]
                  n53 = call <vilib>:"H5Gclose.vi"("error in (no error)"=w321, "group in"=w318) -> ("error out"=w313:errorcluster)  [unwired: 9 in]
                  n54 = xnode "H5Dread.xnode"("dataset name (this)"="IRF Array Time Axis" ("dataset name"), "error in (no error)"=w313, "default"=w350, "ref in"=w304) -> ("error out"=w353:errorcluster, "data"=w329:dbl[], "ref out"=w352:T28)  [unwired: 2 in, 1 out]
                  n55 = xnode "H5Dread.xnode"("dataset name (this)"="IRF Array" ("dataset name"), "error in (no error)"=w353, "default"=w348, "ref in"=w352) -> ("error out"=w284:errorcluster, "data"=w346:dbl[][], "ref out"=w345:T28)  [unwired: 2 in, 1 out]
                  n56 = xnode "H5Dread.xnode"("dataset name (this)"=w289, "error in (no error)"=w284, "default"=w295, "ref in"=w345) -> ("error out"=w285:errorcluster, "data"=w283:T14[], "ref out"=w290:i64)  [unwired: 2 in, 1 out]
                  n57 = case shown="Error .." w285 {
                    selector: w285 -> [w356 _]
                    tunnel: [w355 w365] -> w293
                    tunnel: [w356 w364] -> w292
                    tunnel: [w354 w362] -> w291
                    tunnel: w290 -> [w355 w359]
                    tunnel: w289 -> [_ w358]
                    tunnel: w284 -> [_ w357]
                    tunnel: w283 -> [w354 _]
                    frame No Error {
                      # "New version"
                    }
                    frame Error {
                      # "version 1"
                      n58 = xnode "H5Dread.xnode"("dataset name (this)"=w358, "error in (no error)"=w357, "default"=u16[] [], "ref in"=w359) -> ("error out"=w364:errorcluster, "data"=w361:u16[], "ref out"=w365:i64)  [unwired: 2 in, 1 out]
                      n59 = Array Size(array=w361) -> (size(s)=w360:i32)
                      n60 = call "Get Valid Decay Fit Parameters List.vi"("Parameter ID Array Size"=w360) -> ("Parameter Name Array"=w362:T14[])
                    }
                  }
                  n61 = case shown="No Error" w292 {
                    selector: w292 -> [w382 _]
                    tunnel: w293 -> [w383 w392]
                    tunnel: [w383 w391] -> w286
                    tunnel: [w382 w390] -> w287
                    tunnel: w291 -> [w381 _]
                    tunnel: [w381 w389] -> w282
                    tunnel: "Decay Fit Parameter Names" ("name") -> [_ w385]
                    tunnel: w284 -> [_ w384]
                    frame No Error {
                      # "New version"
                    }
                    frame Error {
                      # "Old version"
                      n62 = xnode "H5Dread.xnode"("dataset name (this)"=w385, "error in (no error)"=w384, "default"=u16[] [], "ref in"=w392) -> ("error out"=w390:errorcluster, "data"=w387:u16[], "ref out"=w391:i64)  [unwired: 2 in, 1 out]
                      n63 = Array Size(array=w387) -> (size(s)=w386:i32)
                      n64 = call "Get Valid Decay Fit Parameters List.vi"("Parameter ID Array Size"=w386) -> ("Parameter Name Array"=w389:T14[])
                    }
                  }
                  n65 = for {
                    tunnel: w334 -> [w485]
                    tunnel: [w484] -> w333 mode=indexing
                    tunnel: w282 -> [w483] mode=indexing
                    n66 = Index Array(array=w485, index=w483) -> (element=w484:string)
                  }
                  n67 = xnode "H5Dread.xnode"("dataset name (this)"="Multiple Decay Fit Parameters Array" ("name"), "error in (no error)"=w287, "default"=w297, "ref in"=w286) -> ("error out"=w303:errorcluster, "data"=w298:dbl[][], "ref out"=w301:T28)  [unwired: 2 in, 1 out]
                  n68 = call "Convert Decay Fit Options v1 to v2.vi"("Decay Fit Options v1"=w280) -> ("Decay Fit Options v2"=w279:T25)
                  n69 = xnode "H5Dread.xnode"("dataset name (this)"="Multiple Decay Fit Parameters SDV Array" ("name"), "error in (no error)"=w303, "default"=w297, "ref in"=w301) -> ("error out"=w302:errorcluster, "data"=w296:dbl[][], "ref out"=w300:T28)  [unwired: 2 in, 1 out]
                  n70 = call "Convert Decay Fit Options v2 to v3.vi"("Decay Fit Options v2"=w279) -> ("Decay Fit Options v3"=w278:T27)
                  n71 = Array Size(array=w298) -> (size(s)=w328:i32[])
                  n72 = Bundle By Name(cluster=w294, "[Multiple Decays Fit Parameters]"=w298, "[Decay Fit Parameter Names]"=w282, "[IRFs]"=w346, "IRF Array Time Axis"=w329) -> (w343:T13)
                  n73 = call "Concatenate String Array.vi"("Separator (TAB)"=", ", "String Array"=w333) -> ("Formatted String"=w331:string)  [unwired: 9 in]
                  n74 = call "AlliGator Convert Decay Fit Options v3 to v4.vi"("Decay Fit Options (v3)"=w278) -> ("Decay Fit Options (v4)"=w277:T2)
                  n75 = Array Size(array=w329) -> (size(s)=w330:i32)
                  n76 = Index Array(array=w328) -> (element #1=w327:i32, element #2=w326:i32)  [unwired: 2 in]
                  n77 = Bundle By Name(cluster=w281, "Fit Parameter Constraints"=w307, "Fit Options"=w277, "SYNC Period"=w306) -> (w305:T1)
                  n78 = Format Into String(format string="Parameter Names: %s\nIRFs Length: %d\n# Data Points: %d x %d", initial string=w336, error in=w302, w331, w330, w327, w326) -> (resulting string=w337:string, error out=w338:errorcluster)
                }
                frame "0.3" {
                  w541 = "Decay Fit Parameter IDs" ("name")
                  # "Was Decay Fit Parameter Names previously"
                  n79 = call "AlliGator Read IRFs & Fit Data HDF5 File Metadata.vi"("error in (no error)"=w611, "ref in"=w612) -> ("error out"=w609:errorcluster, "File Metadata"=w606:string, "ref out"=w610:T28)  [unwired: 7 in]
                  n80 = Unbundle By Name(T23 {"IRF Array Time Axis"=[], "[IRFs]"=[], "[Decay Fit Parameter Names]"=[], "[Multiple Decays Fit Parameters]"=[], "Fit Options: Decay Preprocessing Parameters"={"Background Subtraction"=FALSE, "Straighten Decay"=FALSE, "Reverse Gates"=FALSE, "1-Normalized Decay"=FALSE, "Smoothen Decay"=FALSE, "Smoothing Parameter"=0.0, "Shift Decay"=FALSE, "Decay Shift Parameters"={"Type"=enum."Default", "Shift"=0.0, "Threshold"=0.0, "Rotate"=FALSE}, "Extrapolate Decay"=FALSE, "Additional Points"=0, "Head Fraction"=0.0, "Pixel-Normalize Decay"=FALSE, "Use Periodicity"=FALSE, "Use Cursors"=FALSE, "Tail Fraction"=0.0, "Use Decay Pre-Processing"=FALSE, "Fold Decay"=FALSE, "# Folds"=0, "[0-1]-Normalized Decay"=FALSE}, "Fit Options: Reference Decay"={"t Array"=[], "I Array"=[]}} ("IRFs & Fit Data Map")) -> ("[Multiple Decays Fit Parameters]"=w568:dbl[][], "[Decay Fit Parameter Names]"=w562:T14[], "[IRFs]"=w618:dbl[][], "IRF Array Time Axis"=w620:dbl[], "Fit Options: Decay Preprocessing Parameters"=w549:T15, "Fit Options: Reference Decay"=w547:cluster{"t Array":dbl[], "I Array":dbl[]})
                  n81 = Unbundle By Name(T18 {"SYNC Period"=0.0, "Fit Options"={"Show Fit Residuals"=FALSE, "Fit Model"=enum."1-Exponential", "Residual Type"=enum."Standard", "Max Decay Percentile"=0.0, "Min Decay Percentile"=0.0, "Show Full Decay"=FALSE, "Weights"=enum."Unweighted", "Fitting Method"=enum."Least Square", "Compute Parameter Uncertainties"=FALSE, "Periodic Boundaries"=FALSE, "Model Calculation"=enum."Simulation", "Period"=0.0, "Termination Criteria"={"Max Iterations"=0, "Max Function Calls"=0, "Max Time"=0.0, "Function Tolerance"=0.0, "Parameter Tolerance"=0.0, "Gradient Tolerance"=0.0, "Min Lambda"=0.0, "Max Lambda"=0.0, "Initial Tick Count"=0}, "Offset Resolution"=0.0, "Use Local IRF"=FALSE, "Fitting Algorithm"=enum."Levenberg-Marquardt"}, "Fit Parameter Constraints"=[]} ("Decay Fit Options & Parameters")) -> ("Fit Parameter Constraints"=w579:T9[], "Fit Options"=w580:T19, "SYNC Period"=w581:dbl[unit])
                  n82 = call <vilib>:"H5Gclose.vi"("error in (no error)"=w609, "group in"=w610) -> ("error out"=w584:errorcluster)  [unwired: 9 in]
                  n83 = call <vilib>:"H5Gopen.vi"("error in (no error)"=w584, "name"="Decay Fit Options & Parameters" ("dataset name"), "ref in"=w573) -> ("error out"=w595:errorcluster, "group out"=w594:T28)  [unwired: 7 in]
                  n84 = xnode "H5Dread.xnode"("dataset name (this)"="Laser Period" ("dataset name"), "error in (no error)"=w595, "default"=w581, "ref in"=w594) -> ("error out"=w593:errorcluster, "data"=w575:dbl[unit], "ref out"=w590:T28)  [unwired: 2 in, 1 out]
                  n85 = xnode "H5Dread.xnode"("dataset name (this)"="Fit Options" ("dataset name"), "error in (no error)"=w593, "default"=w580, "ref in"=w590) -> ("error out"=w592:errorcluster, "data"=w576:T19, "ref out"=w589:T28)  [unwired: 2 in, 1 out]
                  n86 = xnode "H5Dread.xnode"("dataset name (this)"="Fit Parameter Constraints" ("dataset name"), "error in (no error)"=w592, "default"=w579, "ref in"=w589) -> ("error out"=w591:errorcluster, "data"=w577:T9[], "ref out"=w588:T28)  [unwired: 2 in, 1 out]
                  n87 = Unbundle By Name(w547) -> ("t Array"=w546:dbl[], "I Array"=w544:dbl[])
                  n88 = call <vilib>:"H5Gclose.vi"("error in (no error)"=w591, "group in"=w588) -> ("error out"=w583:errorcluster)  [unwired: 9 in]
                  n89 = xnode "H5Dread.xnode"("dataset name (this)"="IRF Array Time Axis" ("dataset name"), "error in (no error)"=w583, "default"=w620, "ref in"=w573) -> ("error out"=w623:errorcluster, "data"=w599:dbl[], "ref out"=w622:T28)  [unwired: 2 in, 1 out]
                  n90 = xnode "H5Dread.xnode"("dataset name (this)"="IRF Array" ("dataset name"), "error in (no error)"=w623, "default"=w618, "ref in"=w622) -> ("error out"=w536:errorcluster, "data"=w616:dbl[][], "ref out"=w615:T28)  [unwired: 2 in, 1 out]
                  n91 = xnode "H5Dread.xnode"("dataset name (this)"=w541, "error in (no error)"=w536, "default"=w562, "ref in"=w615) -> ("error out"=w542:errorcluster, "data"=w539:T14[], "ref out"=w538:T28)  [unwired: 2 in, 1 out]
                  n92 = case shown="Error .." w542 {
                    selector: w542 -> [w625 _]
                    tunnel: w538 -> [w626 w631]
                    tunnel: [w626 w635] -> w540
                    tunnel: [w625 w633] -> w537
                    tunnel: [w624 w629] -> w535
                    tunnel: w541 -> [_ w634]
                    tunnel: w536 -> [_ w632]
                    tunnel: w539 -> [w624 _]
                    frame No Error {
                      # "New version"
                    }
                    frame Error {
                      # "version 1"
                      n93 = xnode "H5Dread.xnode"("dataset name (this)"=w634, "error in (no error)"=w632, "default"=u16[] [], "ref in"=w631) -> ("error out"=w633:errorcluster, "data"=w628:u16[], "ref out"=w635:i64)  [unwired: 2 in, 1 out]
                      n94 = Array Size(array=w628) -> (size(s)=w627:i32)
                      n95 = call "Get Valid Decay Fit Parameters List.vi"("Parameter ID Array Size"=w627) -> ("Parameter Name Array"=w629:T14[])
                    }
                  }
                  n96 = case shown="Error .." w537 {
                    selector: w537 -> [w697 _]
                    tunnel: w540 -> [w698 w707]
                    tunnel: [w698 w706] -> w566
                    tunnel: [w697 w704] -> w565
                    tunnel: w535 -> [w696 _]
                    tunnel: [w696 w702] -> w564
                    tunnel: "Decay Fit Parameter Names" ("name") -> [_ w705]
                    tunnel: w536 -> [_ w703]
                    frame No Error {
                      # "New version"
                    }
                    frame Error {
                      # "Old version"
                      n97 = xnode "H5Dread.xnode"("dataset name (this)"=w705, "error in (no error)"=w703, "default"=u16[] [], "ref in"=w707) -> ("error out"=w704:errorcluster, "data"=w700:u16[], "ref out"=w706:i64)  [unwired: 2 in, 1 out]
                      n98 = Array Size(array=w700) -> (size(s)=w699:i32)
                      n99 = call "Get Valid Decay Fit Parameters List.vi"("Parameter ID Array Size"=w699) -> ("Parameter Name Array"=w702:T14[])
                    }
                  }
                  n100 = for {
                    tunnel: w564 -> [w784] mode=indexing
                    tunnel: w604 -> [w785]
                    tunnel: [w783] -> w603 mode=indexing
                    n101 = Index Array(array=w785, index=w784) -> (element=w783:string)
                  }
                  n102 = xnode "H5Dread.xnode"("dataset name (this)"="Multiple Decay Fit Parameters Array" ("name"), "error in (no error)"=w565, "default"=w568, "ref in"=w566) -> ("error out"=w559:errorcluster, "data"=w569:dbl[][], "ref out"=w560:T28)  [unwired: 2 in, 1 out]
                  n103 = xnode "H5Dread.xnode"("dataset name (this)"="Decay Preprocessing Parameters" ("name"), "error in (no error)"=w559, "default"=w549, "ref in"=w560) -> ("error out"=w555:errorcluster, "data"=w548:T15, "ref out"=w558:i64)  [unwired: 2 in, 1 out]
                  n104 = xnode "H5Dread.xnode"("dataset name (this)"="Reference Decay: t Array" ("name"), "error in (no error)"=w555, "default"=w546, "ref in"=w558) -> ("error out"=w554:errorcluster, "data"=w545:dbl[], "ref out"=w557:T28)  [unwired: 2 in, 1 out]
                  n105 = xnode "H5Dread.xnode"("dataset name (this)"="Reference Decay: I Array" ("name"), "error in (no error)"=w554, "default"=w544, "ref in"=w557) -> ("error out"=w553:errorcluster, "data"=w543:dbl[], "ref out"=w556:T28)  [unwired: 2 in, 1 out]
                  n106 = Bundle By Name(cluster=w561, "[Multiple Decays Fit Parameters]"=w569, "[Decay Fit Parameter Names]"=w564, "[IRFs]"=w616, "IRF Array Time Axis"=w599, "Fit Options: Decay Preprocessing Parameters"=w548, "Fit Options: Reference Decay.t Array"=w545, "Fit Options: Reference Decay.I Array"=w543) -> (w613:T13)
                  n107 = call "Convert Decay Fit Options v1 to v2.vi"("Decay Fit Options v1"=w576) -> ("Decay Fit Options v2"=w533:T25)
                  n108 = Array Size(array=w569) -> (size(s)=w598:i32[])
                  n109 = call "Concatenate String Array.vi"("Separator (TAB)"=", ", "String Array"=w603) -> ("Formatted String"=w601:string)  [unwired: 9 in]
                  n110 = xnode "H5Dread.xnode"("dataset name (this)"="Multiple Decay Fit Parameters SDV Array" ("name"), "error in (no error)"=w553, "default"=w568, "ref in"=w556) -> ("error out"=w572:errorcluster, "data"=w567:dbl[][], "ref out"=w571:T28)  [unwired: 2 in, 1 out]
                  n111 = call "Convert Decay Fit Options v2 to v3.vi"("Decay Fit Options v2"=w533) -> ("Decay Fit Options v3"=w532:T27)
                  n112 = Array Size(array=w599) -> (size(s)=w600:i32)
                  n113 = call "AlliGator Convert Decay Fit Options v3 to v4.vi"("Decay Fit Options (v3)"=w532) -> ("Decay Fit Options (v4)"=w531:T2)
                  n114 = Index Array(array=w598) -> (element #1=w597:i32, element #2=w596:i32)  [unwired: 2 in]
                  n115 = Bundle By Name(cluster=w534, "Fit Parameter Constraints"=w577, "Fit Options"=w531, "SYNC Period"=w575) -> (w574:T1)
                  n116 = Format Into String(format string="Parameter Names: %s\nIRFs Length: %d\n# Data Points: %d x %d", initial string=w606, error in=w572, w601, w600, w597, w596) -> (resulting string=w607:string, error out=w608:errorcluster)
                }
                frame "0.4" {
                  w866 = "Decay Fit Parameter IDs" ("name")
                  # "Was Decay Fit Parameter Names previously"
                  n117 = call "AlliGator Read IRFs & Fit Data HDF5 File Metadata.vi"("error in (no error)"=w934, "ref in"=w935) -> ("error out"=w932:errorcluster, "File Metadata"=w929:string, "ref out"=w933:T28)  [unwired: 7 in]
                  n118 = Unbundle By Name(T24 {"SYNC Period"=0.0, "Fit Options"={"Show Fit Residuals"=FALSE, "Fit Model"=enum."1-Exponential", "Residual Type"=enum."Standard", "Max Decay Percentile"=0.0, "Min Decay Percentile"=0.0, "Show Full Decay"=FALSE, "Weights"=enum."Unweighted", "Fitting Method"=enum."Least Square", "Compute Parameter Uncertainties"=FALSE, "Periodic Boundaries"=FALSE, "Model Calculation"=enum."Simulation", "Period"=0.0, "Termination Criteria"={"Max Iterations"=0, "Max Function Calls"=0, "Max Time"=0.0, "Function Tolerance"=0.0, "Parameter Tolerance"=0.0, "Gradient Tolerance"=0.0, "Min Lambda"=0.0, "Max Lambda"=0.0, "Initial Tick Count"=0}, "Offset Resolution"=0.0, "Use Local IRF"=FALSE, "Fitting Algorithm"=enum."Levenberg-Marquardt"}, "Fit Parameter Constraints"=[], "MLE Baseline Offset"=0.0, "MLE Baseline Offset Type"=enum."Absolute"} ("Decay Fit Options & Parameters")) -> ("Fit Parameter Constraints"=w904:T9[], "Fit Options"=w905:T25, "SYNC Period"=w906:dbl[unit], "MLE Baseline Offset Type"=w856:T11, "MLE Baseline Offset"=w850:dbl)
                  n119 = Unbundle By Name(T23 {"IRF Array Time Axis"=[], "[IRFs]"=[], "[Decay Fit Parameter Names]"=[], "[Multiple Decays Fit Parameters]"=[], "Fit Options: Decay Preprocessing Parameters"={"Background Subtraction"=FALSE, "Straighten Decay"=FALSE, "Reverse Gates"=FALSE, "1-Normalized Decay"=FALSE, "Smoothen Decay"=FALSE, "Smoothing Parameter"=0.0, "Shift Decay"=FALSE, "Decay Shift Parameters"={"Type"=enum."Default", "Shift"=0.0, "Threshold"=0.0, "Rotate"=FALSE}, "Extrapolate Decay"=FALSE, "Additional Points"=0, "Head Fraction"=0.0, "Pixel-Normalize Decay"=FALSE, "Use Periodicity"=FALSE, "Use Cursors"=FALSE, "Tail Fraction"=0.0, "Use Decay Pre-Processing"=FALSE, "Fold Decay"=FALSE, "# Folds"=0, "[0-1]-Normalized Decay"=FALSE}, "Fit Options: Reference Decay"={"t Array"=[], "I Array"=[]}} ("IRFs & Fit Data Map")) -> ("[Multiple Decays Fit Parameters]"=w893:dbl[][], "[Decay Fit Parameter Names]"=w887:T14[], "[IRFs]"=w941:dbl[][], "IRF Array Time Axis"=w943:dbl[], "Fit Options: Decay Preprocessing Parameters"=w874:T15, "Fit Options: Reference Decay"=w872:cluster{"t Array":dbl[], "I Array":dbl[]})
                  n120 = call <vilib>:"H5Gclose.vi"("error in (no error)"=w932, "group in"=w933) -> ("error out"=w909:errorcluster)  [unwired: 9 in]
                  n121 = call <vilib>:"H5Gopen.vi"("error in (no error)"=w909, "name"="Decay Fit Options & Parameters" ("dataset name"), "ref in"=w898) -> ("error out"=w918:errorcluster, "group out"=w917:T28)  [unwired: 7 in]
                  n122 = xnode "H5Dread.xnode"("dataset name (this)"="Laser Period" ("dataset name"), "error in (no error)"=w918, "default"=w906, "ref in"=w917) -> ("error out"=w858:errorcluster, "data"=w900:dbl[unit], "ref out"=w855:T28)  [unwired: 2 in, 1 out]
                  n123 = xnode "H5Dread.xnode"("dataset name (this)"="MLE Baseline Offset Type" ("dataset name"), "error in (no error)"=w858, "default"=w856, "ref in"=w855) -> ("error out"=w854:errorcluster, "data"=w849:T11)  [unwired: 2 in, 2 out]
                  n124 = xnode "H5Dread.xnode"("dataset name (this)"="MLE Baseline Offset" ("dataset name"), "error in (no error)"=w854, "default"=w850, "ref in"=w855) -> ("error out"=w852:errorcluster, "data"=w848:dbl, "ref out"=w853:i64)  [unwired: 2 in, 1 out]
                  n125 = xnode "H5Dread.xnode"("dataset name (this)"="Fit Options" ("dataset name"), "error in (no error)"=w852, "default"=w905, "ref in"=w853) -> ("error out"=w916:errorcluster, "data"=w901:T25, "ref out"=w914:T28)  [unwired: 2 in, 1 out]
                  n126 = xnode "H5Dread.xnode"("dataset name (this)"="Fit Parameter Constraints" ("dataset name"), "error in (no error)"=w916, "default"=w904, "ref in"=w914) -> ("error out"=w915:errorcluster, "data"=w902:T9[], "ref out"=w913:T28)  [unwired: 2 in, 1 out]
                  n127 = Unbundle By Name(w872) -> ("t Array"=w871:dbl[], "I Array"=w869:dbl[])
                  n128 = call <vilib>:"H5Gclose.vi"("error in (no error)"=w915, "group in"=w913) -> ("error out"=w908:errorcluster)  [unwired: 9 in]
                  n129 = xnode "H5Dread.xnode"("dataset name (this)"="IRF Array Time Axis" ("dataset name"), "error in (no error)"=w908, "default"=w943, "ref in"=w898) -> ("error out"=w946:errorcluster, "data"=w922:dbl[], "ref out"=w945:T28)  [unwired: 2 in, 1 out]
                  n130 = xnode "H5Dread.xnode"("dataset name (this)"="IRF Array" ("dataset name"), "error in (no error)"=w946, "default"=w941, "ref in"=w945) -> ("error out"=w861:errorcluster, "data"=w939:dbl[][], "ref out"=w938:T28)  [unwired: 2 in, 1 out]
                  n131 = xnode "H5Dread.xnode"("dataset name (this)"=w866, "error in (no error)"=w861, "default"=w887, "ref in"=w938) -> ("error out"=w867:errorcluster, "data"=w864:T14[], "ref out"=w863:T28)  [unwired: 2 in, 1 out]
                  n132 = case shown="Error .." w867 {
                    selector: w867 -> [w978 _]
                    tunnel: w863 -> [w979 w984]
                    tunnel: [w979 w988] -> w865
                    tunnel: [w978 w986] -> w862
                    tunnel: [w977 w982] -> w860
                    tunnel: w866 -> [_ w987]
                    tunnel: w861 -> [_ w985]
                    tunnel: w864 -> [w977 _]
                    frame No Error {
                      # "New version"
                    }
                    frame Error {
                      # "version 1"
                      n133 = xnode "H5Dread.xnode"("dataset name (this)"=w987, "error in (no error)"=w985, "default"=u16[] [], "ref in"=w984) -> ("error out"=w986:errorcluster, "data"=w981:u16[], "ref out"=w988:i64)  [unwired: 2 in, 1 out]
                      n134 = Array Size(array=w981) -> (size(s)=w980:i32)
                      n135 = call "Get Valid Decay Fit Parameters List.vi"("Parameter ID Array Size"=w980) -> ("Parameter Name Array"=w982:T14[])
                    }
                  }
                  n136 = case shown="Error .." w862 {
                    selector: w862 -> [w1050 _]
                    tunnel: w865 -> [w1051 w1060]
                    tunnel: [w1051 w1059] -> w891
                    tunnel: [w1050 w1057] -> w890
                    tunnel: w860 -> [w1049 _]
                    tunnel: [w1049 w1055] -> w889
                    tunnel: "Decay Fit Parameter Names" ("name") -> [_ w1058]
                    tunnel: w861 -> [_ w1056]
                    frame No Error {
                      # "New version"
                    }
                    frame Error {
                      # "Old version"
                      n137 = xnode "H5Dread.xnode"("dataset name (this)"=w1058, "error in (no error)"=w1056, "default"=u16[] [], "ref in"=w1060) -> ("error out"=w1057:errorcluster, "data"=w1053:u16[], "ref out"=w1059:i64)  [unwired: 2 in, 1 out]
                      n138 = Array Size(array=w1053) -> (size(s)=w1052:i32)
                      n139 = call "Get Valid Decay Fit Parameters List.vi"("Parameter ID Array Size"=w1052) -> ("Parameter Name Array"=w1055:T14[])
                    }
                  }
                  n140 = for {
                    tunnel: w889 -> [w1137] mode=indexing
                    tunnel: w927 -> [w1138]
                    tunnel: [w1136] -> w926 mode=indexing
                    n141 = Index Array(array=w1138, index=w1137) -> (element=w1136:string)
                  }
                  n142 = xnode "H5Dread.xnode"("dataset name (this)"="Multiple Decay Fit Parameters Array" ("name"), "error in (no error)"=w890, "default"=w893, "ref in"=w891) -> ("error out"=w884:errorcluster, "data"=w894:dbl[][], "ref out"=w885:T28)  [unwired: 2 in, 1 out]
                  n143 = xnode "H5Dread.xnode"("dataset name (this)"="Decay Preprocessing Parameters" ("name"), "error in (no error)"=w884, "default"=w874, "ref in"=w885) -> ("error out"=w880:errorcluster, "data"=w873:T15, "ref out"=w883:T28)  [unwired: 2 in, 1 out]
                  n144 = xnode "H5Dread.xnode"("dataset name (this)"="Reference Decay: t Array" ("name"), "error in (no error)"=w880, "default"=w871, "ref in"=w883) -> ("error out"=w879:errorcluster, "data"=w870:dbl[], "ref out"=w882:T28)  [unwired: 2 in, 1 out]
                  n145 = xnode "H5Dread.xnode"("dataset name (this)"="Reference Decay: I Array" ("name"), "error in (no error)"=w879, "default"=w869, "ref in"=w882) -> ("error out"=w878:errorcluster, "data"=w868:dbl[], "ref out"=w881:T28)  [unwired: 2 in, 1 out]
                  n146 = Bundle By Name(cluster=w886, "[Multiple Decays Fit Parameters]"=w894, "[Decay Fit Parameter Names]"=w889, "[IRFs]"=w939, "IRF Array Time Axis"=w922, "Fit Options: Decay Preprocessing Parameters"=w873, "Fit Options: Reference Decay.t Array"=w870, "Fit Options: Reference Decay.I Array"=w868) -> (w936:T13)
                  n147 = Array Size(array=w894) -> (size(s)=w921:i32[])
                  n148 = call "Convert Decay Fit Options v2 to v3.vi"("Decay Fit Options v2"=w901) -> ("Decay Fit Options v3"=w847:T27)
                  n149 = call "Concatenate String Array.vi"("Separator (TAB)"=", ", "String Array"=w926) -> ("Formatted String"=w924:string)  [unwired: 9 in]
                  n150 = xnode "H5Dread.xnode"("dataset name (this)"="Multiple Decay Fit Parameters SDV Array" ("name"), "error in (no error)"=w878, "default"=w893, "ref in"=w881) -> ("error out"=w897:errorcluster, "data"=w892:dbl[][], "ref out"=w896:T28)  [unwired: 2 in, 1 out]
                  n151 = call "AlliGator Convert Decay Fit Options v3 to v4.vi"("Decay Fit Options (v3)"=w847) -> ("Decay Fit Options (v4)"=w846:T2)
                  n152 = Array Size(array=w922) -> (size(s)=w923:i32)
                  n153 = Index Array(array=w921) -> (element #1=w920:i32, element #2=w919:i32)  [unwired: 2 in]
                  n154 = Bundle By Name(cluster=w859, "Fit Parameter Constraints"=w902, "Fit Options"=w846, "SYNC Period"=w900, "MLE Baseline Offset Type"=w849, "MLE Baseline Offset"=w848) -> (w899:T1)
                  n155 = Format Into String(format string="Parameter Names: %s\nIRFs Length: %d\n# Data Points: %d x %d", initial string=w929, error in=w897, w924, w923, w920, w919) -> (resulting string=w930:string, error out=w931:errorcluster)
                }
                frame "0.5" {
                  w1218 = "Decay Fit Parameter IDs" ("name")
                  # "Was Decay Fit Parameter Names previously"
                  n156 = Unbundle By Name(T26 {"SYNC Period"=0.0, "Fit Options"={"Show Fit Residuals"=FALSE, "Fit Model"=enum."1-Exponential", "Residual Type"=enum."Standard", "Max Decay Percentile"=0.0, "Min Decay Percentile"=0.0, "Show Full Decay"=FALSE, "Weights"=enum."Unweighted", "Fitting Method"=enum."Least Square", "Compute Parameter Uncertainties"=FALSE, "Periodic Boundaries"=FALSE, "Model Calculation"=enum."Simulation", "Period"=0.0, "Termination Criteria"={"Max Iterations"=0, "Max Function Calls"=0, "Max Time"=0.0, "Function Tolerance"=0.0, "Parameter Tolerance"=0.0, "Gradient Tolerance"=0.0, "Min Lambda"=0.0, "Max Lambda"=0.0, "Initial Tick Count"=0}, "Offset Resolution"=0.0, "Use Local IRF"=FALSE, "Fitting Algorithm"=enum."Levenberg-Marquardt", "Show Confidence Interval "=TRUE, "Confidence Level"=95.0}, "Fit Parameter Constraints"=[], "MLE Baseline Offset"=0.0, "MLE Baseline Offset Type"=enum."Absolute"} ("Decay Fit Options & Parameters")) -> ("Fit Parameter Constraints"=w1256:T9[], "Fit Options"=w1257:T27, "SYNC Period"=w1258:dbl[unit], "MLE Baseline Offset Type"=w1208:T11, "MLE Baseline Offset"=w1202:dbl)
                  n157 = call "AlliGator Read IRFs & Fit Data HDF5 File Metadata.vi"("error in (no error)"=w1286, "ref in"=w1287) -> ("error out"=w1284:errorcluster, "File Metadata"=w1281:string, "ref out"=w1285:T28)  [unwired: 7 in]
                  n158 = Unbundle By Name(T23 {"IRF Array Time Axis"=[], "[IRFs]"=[], "[Decay Fit Parameter Names]"=[], "[Multiple Decays Fit Parameters]"=[], "Fit Options: Decay Preprocessing Parameters"={"Background Subtraction"=FALSE, "Straighten Decay"=FALSE, "Reverse Gates"=FALSE, "1-Normalized Decay"=FALSE, "Smoothen Decay"=FALSE, "Smoothing Parameter"=0.0, "Shift Decay"=FALSE, "Decay Shift Parameters"={"Type"=enum."Default", "Shift"=0.0, "Threshold"=0.0, "Rotate"=FALSE}, "Extrapolate Decay"=FALSE, "Additional Points"=0, "Head Fraction"=0.0, "Pixel-Normalize Decay"=FALSE, "Use Periodicity"=FALSE, "Use Cursors"=FALSE, "Tail Fraction"=0.0, "Use Decay Pre-Processing"=FALSE, "Fold Decay"=FALSE, "# Folds"=0, "[0-1]-Normalized Decay"=FALSE}, "Fit Options: Reference Decay"={"t Array"=[], "I Array"=[]}} ("IRFs & Fit Data Map")) -> ("[Multiple Decays Fit Parameters]"=w1245:dbl[][], "[Decay Fit Parameter Names]"=w1239:T14[], "[IRFs]"=w1293:dbl[][], "IRF Array Time Axis"=w1295:dbl[], "Fit Options: Decay Preprocessing Parameters"=w1226:T15, "Fit Options: Reference Decay"=w1224:cluster{"t Array":dbl[], "I Array":dbl[]})
                  n159 = call <vilib>:"H5Gclose.vi"("error in (no error)"=w1284, "group in"=w1285) -> ("error out"=w1261:errorcluster)  [unwired: 9 in]
                  n160 = call <vilib>:"H5Gopen.vi"("error in (no error)"=w1261, "name"="Decay Fit Options & Parameters" ("dataset name"), "ref in"=w1250) -> ("error out"=w1270:errorcluster, "group out"=w1269:T28)  [unwired: 7 in]
                  n161 = xnode "H5Dread.xnode"("dataset name (this)"="Laser Period" ("dataset name"), "error in (no error)"=w1270, "default"=w1258, "ref in"=w1269) -> ("error out"=w1210:errorcluster, "data"=w1252:dbl[unit], "ref out"=w1207:T28)  [unwired: 2 in, 1 out]
                  n162 = xnode "H5Dread.xnode"("dataset name (this)"="MLE Baseline Offset Type" ("dataset name"), "error in (no error)"=w1210, "default"=w1208, "ref in"=w1207) -> ("error out"=w1206:errorcluster, "data"=w1201:T11)  [unwired: 2 in, 2 out]
                  n163 = xnode "H5Dread.xnode"("dataset name (this)"="MLE Baseline Offset" ("dataset name"), "error in (no error)"=w1206, "default"=w1202, "ref in"=w1207) -> ("error out"=w1204:errorcluster, "data"=w1200:dbl, "ref out"=w1205:i64)  [unwired: 2 in, 1 out]
                  n164 = xnode "H5Dread.xnode"("dataset name (this)"="Fit Options" ("dataset name"), "error in (no error)"=w1204, "default"=w1257, "ref in"=w1205) -> ("error out"=w1268:errorcluster, "data"=w1253:T27, "ref out"=w1266:T28)  [unwired: 2 in, 1 out]
                  n165 = xnode "H5Dread.xnode"("dataset name (this)"="Fit Parameter Constraints" ("dataset name"), "error in (no error)"=w1268, "default"=w1256, "ref in"=w1266) -> ("error out"=w1267:errorcluster, "data"=w1254:T9[], "ref out"=w1265:T28)  [unwired: 2 in, 1 out]
                  n166 = Unbundle By Name(w1224) -> ("t Array"=w1223:dbl[], "I Array"=w1221:dbl[])
                  n167 = call <vilib>:"H5Gclose.vi"("error in (no error)"=w1267, "group in"=w1265) -> ("error out"=w1260:errorcluster)  [unwired: 9 in]
                  n168 = xnode "H5Dread.xnode"("dataset name (this)"="IRF Array Time Axis" ("dataset name"), "error in (no error)"=w1260, "default"=w1295, "ref in"=w1250) -> ("error out"=w1298:errorcluster, "data"=w1274:dbl[], "ref out"=w1297:T28)  [unwired: 2 in, 1 out]
                  n169 = xnode "H5Dread.xnode"("dataset name (this)"="IRF Array" ("dataset name"), "error in (no error)"=w1298, "default"=w1293, "ref in"=w1297) -> ("error out"=w1213:errorcluster, "data"=w1291:dbl[][], "ref out"=w1290:T28)  [unwired: 2 in, 1 out]
                  n170 = xnode "H5Dread.xnode"("dataset name (this)"=w1218, "error in (no error)"=w1213, "default"=w1239, "ref in"=w1290) -> ("error out"=w1219:errorcluster, "data"=w1216:T14[], "ref out"=w1215:T28)  [unwired: 2 in, 1 out]
                  n171 = case shown="Error .." w1219 {
                    selector: w1219 -> [w1330 _]
                    tunnel: w1215 -> [w1331 w1336]
                    tunnel: [w1331 w1340] -> w1217
                    tunnel: [w1330 w1338] -> w1214
                    tunnel: [w1329 w1334] -> w1212
                    tunnel: w1218 -> [_ w1339]
                    tunnel: w1213 -> [_ w1337]
                    tunnel: w1216 -> [w1329 _]
                    frame No Error {
                      # "New version"
                    }
                    frame Error {
                      # "version 1"
                      n172 = xnode "H5Dread.xnode"("dataset name (this)"=w1339, "error in (no error)"=w1337, "default"=u16[] [], "ref in"=w1336) -> ("error out"=w1338:errorcluster, "data"=w1333:u16[], "ref out"=w1340:i64)  [unwired: 2 in, 1 out]
                      n173 = Array Size(array=w1333) -> (size(s)=w1332:i32)
                      n174 = call "Get Valid Decay Fit Parameters List.vi"("Parameter ID Array Size"=w1332) -> ("Parameter Name Array"=w1334:T14[])
                    }
                  }
                  n175 = case shown="Error .." w1214 {
                    selector: w1214 -> [w1402 _]
                    tunnel: w1217 -> [w1403 w1412]
                    tunnel: [w1403 w1411] -> w1243
                    tunnel: [w1402 w1409] -> w1242
                    tunnel: w1212 -> [w1401 _]
                    tunnel: [w1401 w1407] -> w1241
                    tunnel: "Decay Fit Parameter Names" ("name") -> [_ w1410]
                    tunnel: w1213 -> [_ w1408]
                    frame No Error {
                      # "New version"
                    }
                    frame Error {
                      # "Old version"
                      n176 = xnode "H5Dread.xnode"("dataset name (this)"=w1410, "error in (no error)"=w1408, "default"=u16[] [], "ref in"=w1412) -> ("error out"=w1409:errorcluster, "data"=w1405:u16[], "ref out"=w1411:i64)  [unwired: 2 in, 1 out]
                      n177 = Array Size(array=w1405) -> (size(s)=w1404:i32)
                      n178 = call "Get Valid Decay Fit Parameters List.vi"("Parameter ID Array Size"=w1404) -> ("Parameter Name Array"=w1407:T14[])
                    }
                  }
                  n179 = for {
                    tunnel: w1241 -> [w1489] mode=indexing
                    tunnel: w1279 -> [w1490]
                    tunnel: [w1488] -> w1278 mode=indexing
                    n180 = Index Array(array=w1490, index=w1489) -> (element=w1488:string)
                  }
                  n181 = xnode "H5Dread.xnode"("dataset name (this)"="Multiple Decay Fit Parameters Array" ("name"), "error in (no error)"=w1242, "default"=w1245, "ref in"=w1243) -> ("error out"=w1236:errorcluster, "data"=w1246:dbl[][], "ref out"=w1237:T28)  [unwired: 2 in, 1 out]
                  n182 = xnode "H5Dread.xnode"("dataset name (this)"="Decay Preprocessing Parameters" ("name"), "error in (no error)"=w1236, "default"=w1226, "ref in"=w1237) -> ("error out"=w1232:errorcluster, "data"=w1225:T15, "ref out"=w1235:T28)  [unwired: 2 in, 1 out]
                  n183 = xnode "H5Dread.xnode"("dataset name (this)"="Reference Decay: t Array" ("name"), "error in (no error)"=w1232, "default"=w1223, "ref in"=w1235) -> ("error out"=w1231:errorcluster, "data"=w1222:dbl[], "ref out"=w1234:T28)  [unwired: 2 in, 1 out]
                  n184 = xnode "H5Dread.xnode"("dataset name (this)"="Reference Decay: I Array" ("name"), "error in (no error)"=w1231, "default"=w1221, "ref in"=w1234) -> ("error out"=w1230:errorcluster, "data"=w1220:dbl[], "ref out"=w1233:T28)  [unwired: 2 in, 1 out]
                  n185 = Bundle By Name(cluster=w1238, "[Multiple Decays Fit Parameters]"=w1246, "[Decay Fit Parameter Names]"=w1241, "[IRFs]"=w1291, "IRF Array Time Axis"=w1274, "Fit Options: Decay Preprocessing Parameters"=w1225, "Fit Options: Reference Decay.t Array"=w1222, "Fit Options: Reference Decay.I Array"=w1220) -> (w1288:T13)
                  n186 = call "AlliGator Convert Decay Fit Options v3 to v4.vi"("Decay Fit Options (v3)"=w1253) -> ("Decay Fit Options (v4)"=w1199:T2)
                  n187 = Array Size(array=w1246) -> (size(s)=w1273:i32[])
                  n188 = call "Concatenate String Array.vi"("Separator (TAB)"=", ", "String Array"=w1278) -> ("Formatted String"=w1276:string)  [unwired: 9 in]
                  n189 = xnode "H5Dread.xnode"("dataset name (this)"="Multiple Decay Fit Parameters SDV Array" ("name"), "error in (no error)"=w1230, "default"=w1245, "ref in"=w1233) -> ("error out"=w1249:errorcluster, "data"=w1244:dbl[][], "ref out"=w1248:T28)  [unwired: 2 in, 1 out]
                  n190 = Array Size(array=w1274) -> (size(s)=w1275:i32)
                  n191 = Index Array(array=w1273) -> (element #1=w1272:i32, element #2=w1271:i32)  [unwired: 2 in]
                  n192 = Bundle By Name(cluster=w1211, "Fit Parameter Constraints"=w1254, "Fit Options"=w1199, "SYNC Period"=w1252, "MLE Baseline Offset Type"=w1201, "MLE Baseline Offset"=w1200) -> (w1251:T1)
                  n193 = Format Into String(format string="Parameter Names: %s\nIRFs Length: %d\n# Data Points: %d x %d", initial string=w1281, error in=w1249, w1276, w1275, w1272, w1271) -> (resulting string=w1282:string, error out=w1283:errorcluster)
                }
                frame "0.6" {
                  w1577 = "Decay Fit Parameter IDs" ("name")
                  # "Was Decay Fit Parameter Names previously"
                  n194 = Unbundle By Name(T26 {"SYNC Period"=0.0, "Fit Options"={"Show Fit Residuals"=FALSE, "Fit Model"=enum."1-Exponential", "Residual Type"=enum."Standard", "Max Decay Percentile"=0.0, "Min Decay Percentile"=0.0, "Show Full Decay"=FALSE, "Weights"=enum."Unweighted", "Fitting Method"=enum."Least Square", "Compute Parameter Uncertainties"=FALSE, "Periodic Boundaries"=FALSE, "Model Calculation"=enum."Simulation", "Period"=0.0, "Termination Criteria"={"Max Iterations"=0, "Max Function Calls"=0, "Max Time"=0.0, "Function Tolerance"=0.0, "Parameter Tolerance"=0.0, "Gradient Tolerance"=0.0, "Min Lambda"=0.0, "Max Lambda"=0.0, "Initial Tick Count"=0}, "Offset Resolution"=0.0, "Use Local IRF"=FALSE, "Fitting Algorithm"=enum."Levenberg-Marquardt", "Show Confidence Interval "=TRUE, "Confidence Level"=95.0}, "Fit Parameter Constraints"=[], "MLE Baseline Offset"=0.0, "MLE Baseline Offset Type"=enum."Absolute"} ("Decay Fit Options & Parameters")) -> ("Fit Parameter Constraints"=w1613:T9[], "Fit Options"=w1614:T27, "SYNC Period"=w1615:dbl[unit], "MLE Baseline Offset Type"=w1567:T11, "MLE Baseline Offset"=w1561:dbl)
                  n195 = call "AlliGator Read IRFs & Fit Data HDF5 File Metadata.vi"("error in (no error)"=w1643, "ref in"=w1644) -> ("error out"=w1641:errorcluster, "File Metadata"=w1638:string, "ref out"=w1642:T28)  [unwired: 7 in]
                  n196 = Unbundle By Name(T13 {"IRF Array Time Axis"=[], "[IRFs]"=[], "[Decay Fit Parameter Names]"=[], "[Multiple Decays Fit Parameters]"=[], "Fit Options: Decay Preprocessing Parameters"={"Background Subtraction"=FALSE, "Straighten Decay"=FALSE, "Reverse Gates"=FALSE, "1-Normalized Decay"=FALSE, "Smoothen Decay"=FALSE, "Smoothing Parameter"=0.0, "Shift Decay"=FALSE, "Decay Shift Parameters"={"Type"=enum."Default", "Shift"=0.0, "Threshold"=0.0, "Rotate"=FALSE}, "Extrapolate Decay"=FALSE, "Additional Points"=0, "Head Fraction"=0.0, "Pixel-Normalize Decay"=FALSE, "Use Periodicity"=FALSE, "Use Cursors"=FALSE, "Tail Fraction"=0.0, "Use Decay Pre-Processing"=FALSE, "Fold Decay"=FALSE, "# Folds"=0, "[0-1]-Normalized Decay"=FALSE}, "Fit Options: Reference Decay"={"t Array"=[], "I Array"=[]}, "[Decay Sum]"=[]} ("IRFs & Fit Data Map")) -> ("[Multiple Decays Fit Parameters]"=w1602:dbl[][], "[Decay Fit Parameter Names]"=w1596:T14[], "[IRFs]"=w1650:dbl[][], "IRF Array Time Axis"=w1652:dbl[], "Fit Options: Decay Preprocessing Parameters"=w1585:T15, "Fit Options: Reference Decay"=w1583:cluster{"t Array":dbl[], "I Array":dbl[]}, "[Decay Sum]"=w1553:dbl[])
                  n197 = call <vilib>:"H5Gclose.vi"("error in (no error)"=w1641, "group in"=w1642) -> ("error out"=w1618:errorcluster)  [unwired: 9 in]
                  n198 = call <vilib>:"H5Gopen.vi"("error in (no error)"=w1618, "name"="Decay Fit Options & Parameters" ("dataset name"), "ref in"=w1607) -> ("error out"=w1627:errorcluster, "group out"=w1626:T28)  [unwired: 7 in]
                  n199 = xnode "H5Dread.xnode"("dataset name (this)"="Laser Period" ("dataset name"), "error in (no error)"=w1627, "default"=w1615, "ref in"=w1626) -> ("error out"=w1569:errorcluster, "data"=w1609:dbl[unit], "ref out"=w1566:T28)  [unwired: 2 in, 1 out]
                  n200 = xnode "H5Dread.xnode"("dataset name (this)"="MLE Baseline Offset Type" ("dataset name"), "error in (no error)"=w1569, "default"=w1567, "ref in"=w1566) -> ("error out"=w1565:errorcluster, "data"=w1560:T11)  [unwired: 2 in, 2 out]
                  n201 = xnode "H5Dread.xnode"("dataset name (this)"="MLE Baseline Offset" ("dataset name"), "error in (no error)"=w1565, "default"=w1561, "ref in"=w1566) -> ("error out"=w1563:errorcluster, "data"=w1559:dbl, "ref out"=w1564:i64)  [unwired: 2 in, 1 out]
                  n202 = xnode "H5Dread.xnode"("dataset name (this)"="Fit Options" ("dataset name"), "error in (no error)"=w1563, "default"=w1614, "ref in"=w1564) -> ("error out"=w1625:errorcluster, "data"=w1610:T27, "ref out"=w1623:T28)  [unwired: 2 in, 1 out]
                  n203 = xnode "H5Dread.xnode"("dataset name (this)"="Fit Parameter Constraints" ("dataset name"), "error in (no error)"=w1625, "default"=w1613, "ref in"=w1623) -> ("error out"=w1624:errorcluster, "data"=w1611:T9[], "ref out"=w1622:T28)  [unwired: 2 in, 1 out]
                  n204 = Unbundle By Name(w1583) -> ("t Array"=w1582:dbl[], "I Array"=w1580:dbl[])
                  n205 = call <vilib>:"H5Gclose.vi"("error in (no error)"=w1624, "group in"=w1622) -> ("error out"=w1617:errorcluster)  [unwired: 9 in]
                  n206 = xnode "H5Dread.xnode"("dataset name (this)"="IRF Array Time Axis" ("dataset name"), "error in (no error)"=w1617, "default"=w1652, "ref in"=w1607) -> ("error out"=w1655:errorcluster, "data"=w1631:dbl[], "ref out"=w1654:T28)  [unwired: 2 in, 1 out]
                  n207 = xnode "H5Dread.xnode"("dataset name (this)"="IRF Array" ("dataset name"), "error in (no error)"=w1655, "default"=w1650, "ref in"=w1654) -> ("error out"=w1572:errorcluster, "data"=w1648:dbl[][], "ref out"=w1647:T28)  [unwired: 2 in, 1 out]
                  n208 = xnode "H5Dread.xnode"("dataset name (this)"=w1577, "error in (no error)"=w1572, "default"=w1596, "ref in"=w1647) -> ("error out"=w1578:errorcluster, "data"=w1575:T14[], "ref out"=w1574:T28)  [unwired: 2 in, 1 out]
                  n209 = case shown="Error .." w1578 {
                    selector: w1578 -> [w1702 _]
                    tunnel: w1574 -> [w1703 w1708]
                    tunnel: [w1703 w1712] -> w1576
                    tunnel: [w1702 w1710] -> w1573
                    tunnel: [w1701 w1706] -> w1571
                    tunnel: w1577 -> [_ w1711]
                    tunnel: w1572 -> [_ w1709]
                    tunnel: w1575 -> [w1701 _]
                    frame No Error {
                      # "New version"
                    }
                    frame Error {
                      # "version 1"
                      n210 = xnode "H5Dread.xnode"("dataset name (this)"=w1711, "error in (no error)"=w1709, "default"=u16[] [], "ref in"=w1708) -> ("error out"=w1710:errorcluster, "data"=w1705:u16[], "ref out"=w1712:i64)  [unwired: 2 in, 1 out]
                      n211 = Array Size(array=w1705) -> (size(s)=w1704:i32)
                      n212 = call "Get Valid Decay Fit Parameters List.vi"("Parameter ID Array Size"=w1704) -> ("Parameter Name Array"=w1706:T14[])
                    }
                  }
                  n213 = case shown="Error .." w1573 {
                    selector: w1573 -> [w1774 _]
                    tunnel: w1576 -> [w1775 w1784]
                    tunnel: [w1775 w1783] -> w1600
                    tunnel: [w1774 w1781] -> w1599
                    tunnel: w1571 -> [w1773 _]
                    tunnel: [w1773 w1779] -> w1598
                    tunnel: "Decay Fit Parameter Names" ("name") -> [_ w1782]
                    tunnel: w1572 -> [_ w1780]
                    frame No Error {
                      # "New version"
                    }
                    frame Error {
                      # "Old version"
                      n214 = xnode "H5Dread.xnode"("dataset name (this)"=w1782, "error in (no error)"=w1780, "default"=u16[] [], "ref in"=w1784) -> ("error out"=w1781:errorcluster, "data"=w1777:u16[], "ref out"=w1783:i64)  [unwired: 2 in, 1 out]
                      n215 = Array Size(array=w1777) -> (size(s)=w1776:i32)
                      n216 = call "Get Valid Decay Fit Parameters List.vi"("Parameter ID Array Size"=w1776) -> ("Parameter Name Array"=w1779:T14[])
                    }
                  }
                  n217 = for {
                    tunnel: w1598 -> [w1861] mode=indexing
                    tunnel: w1636 -> [w1862]
                    tunnel: [w1860] -> w1635 mode=indexing
                    n218 = Index Array(array=w1862, index=w1861) -> (element=w1860:string)
                  }
                  n219 = xnode "H5Dread.xnode"("dataset name (this)"="Multiple Decay Fit Parameters Array" ("name"), "error in (no error)"=w1599, "default"=w1602, "ref in"=w1600) -> ("error out"=w1593:errorcluster, "data"=w1603:dbl[][], "ref out"=w1594:T28)  [unwired: 2 in, 1 out]
                  n220 = xnode "H5Dread.xnode"("dataset name (this)"="Decay Preprocessing Parameters" ("name"), "error in (no error)"=w1593, "default"=w1585, "ref in"=w1594) -> ("error out"=w1590:errorcluster, "data"=w1584:T15, "ref out"=w1592:T28)  [unwired: 2 in, 1 out]
                  n221 = xnode "H5Dread.xnode"("dataset name (this)"="Reference Decay: t Array" ("name"), "error in (no error)"=w1590, "default"=w1582, "ref in"=w1592) -> ("error out"=w1589:errorcluster, "data"=w1581:dbl[], "ref out"=w1591:T28)  [unwired: 2 in, 1 out]
                  n222 = xnode "H5Dread.xnode"("dataset name (this)"="Reference Decay: I Array" ("name"), "error in (no error)"=w1589, "default"=w1580, "ref in"=w1591) -> ("error out"=w1557:errorcluster, "data"=w1579:dbl[], "ref out"=w1558:T28)  [unwired: 2 in, 1 out]
                  n223 = xnode "H5Dread.xnode"("dataset name (this)"="Decay Sums" ("name"), "error in (no error)"=w1557, "default"=w1553, "ref in"=w1558) -> ("error out"=w1555:errorcluster, "data"=w1552:dbl[], "ref out"=w1556:i64)  [unwired: 2 in, 1 out]
                  n224 = Bundle By Name(cluster=w1595, "[Multiple Decays Fit Parameters]"=w1603, "[Decay Fit Parameter Names]"=w1598, "[IRFs]"=w1648, "IRF Array Time Axis"=w1631, "Fit Options: Decay Preprocessing Parameters"=w1584, "Fit Options: Reference Decay.t Array"=w1581, "Fit Options: Reference Decay.I Array"=w1579, "[Decay Sum]"=w1552) -> (w1645:T13)
                  n225 = Array Size(array=w1603) -> (size(s)=w1630:i32[])
                  n226 = call "AlliGator Convert Decay Fit Options v3 to v4.vi"("Decay Fit Options (v3)"=w1610) -> ("Decay Fit Options (v4)"=w1551:T2)
                  n227 = call "Concatenate String Array.vi"("Separator (TAB)"=", ", "String Array"=w1635) -> ("Formatted String"=w1633:string)  [unwired: 9 in]
                  n228 = xnode "H5Dread.xnode"("dataset name (this)"="Multiple Decay Fit Parameters SDV Array" ("name"), "error in (no error)"=w1555, "default"=w1602, "ref in"=w1556) -> ("error out"=w1606:errorcluster, "data"=w1601:dbl[][], "ref out"=w1605:T28)  [unwired: 2 in, 1 out]
                  n229 = Array Size(array=w1631) -> (size(s)=w1632:i32)
                  n230 = Index Array(array=w1630) -> (element #1=w1629:i32, element #2=w1628:i32)  [unwired: 2 in]
                  n231 = Bundle By Name(cluster=w1570, "Fit Parameter Constraints"=w1611, "Fit Options"=w1551, "SYNC Period"=w1609, "MLE Baseline Offset Type"=w1560, "MLE Baseline Offset"=w1559) -> (w1608:T1)
                  n232 = Format Into String(format string="Parameter Names: %s\nIRFs Length: %d\n# Data Points: %d x %d", initial string=w1638, error in=w1606, w1633, w1632, w1629, w1628) -> (resulting string=w1639:string, error out=w1640:errorcluster)
                }
                frame "0.7" {
                  w1948 = "Decay Fit Parameter IDs" ("name")
                  # "Was Decay Fit Parameter Names previously"
                  n233 = Unbundle By Name(T1 {"SYNC Period"=0.0, "Fit Options"={"Show Fit Residuals"=FALSE, "Fit Model"=enum."1-Exponential", "Residual Type"=enum."Standard", "Max Decay Percentile"=0.0, "Min Decay Percentile"=0.0, "Show Full Decay"=FALSE, "Weights"=enum."Unweighted", "Fitting Method"=enum."Least Square", "Compute Parameter Uncertainties"=FALSE, "Periodic Boundaries"=FALSE, "Model Calculation"=enum."Simulation", "Period"=0.0, "Termination Criteria"={"Max Iterations"=0, "Max Function Calls"=0, "Max Time"=0.0, "Function Tolerance"=0.0, "Parameter Tolerance"=0.0, "Gradient Tolerance"=0.0, "Min Lambda"=0.0, "Max Lambda"=0.0, "Initial Tick Count"=0}, "Offset Resolution"=0.0, "Use Local IRF"=FALSE, "Fitting Algorithm"=enum."Levenberg-Marquardt", "Show Confidence Interval "=TRUE, "Confidence Level"=95.0}, "Fit Parameter Constraints"=[], "MLE Baseline Offset"=0.0, "MLE Baseline Offset Type"=enum."Absolute"} ("Decay Fit Options & Parameters")) -> ("Fit Parameter Constraints"=w1984:T9[], "Fit Options"=w1985:T2, "SYNC Period"=w1986:dbl[unit], "MLE Baseline Offset Type"=w1938:T11, "MLE Baseline Offset"=w1932:dbl)
                  n234 = call "AlliGator Read IRFs & Fit Data HDF5 File Metadata.vi"("error in (no error)"=w2014, "ref in"=w2015) -> ("error out"=w2012:errorcluster, "File Metadata"=w2009:string, "ref out"=w2013:T28)  [unwired: 7 in]
                  n235 = Unbundle By Name(T13 {"IRF Array Time Axis"=[], "[IRFs]"=[], "[Decay Fit Parameter Names]"=[], "[Multiple Decays Fit Parameters]"=[], "Fit Options: Decay Preprocessing Parameters"={"Background Subtraction"=FALSE, "Straighten Decay"=FALSE, "Reverse Gates"=FALSE, "1-Normalized Decay"=FALSE, "Smoothen Decay"=FALSE, "Smoothing Parameter"=0.0, "Shift Decay"=FALSE, "Decay Shift Parameters"={"Type"=enum."Default", "Shift"=0.0, "Threshold"=0.0, "Rotate"=FALSE}, "Extrapolate Decay"=FALSE, "Additional Points"=0, "Head Fraction"=0.0, "Pixel-Normalize Decay"=FALSE, "Use Periodicity"=FALSE, "Use Cursors"=FALSE, "Tail Fraction"=0.0, "Use Decay Pre-Processing"=FALSE, "Fold Decay"=FALSE, "# Folds"=0, "[0-1]-Normalized Decay"=FALSE}, "Fit Options: Reference Decay"={"t Array"=[], "I Array"=[]}, "[Decay Sum]"=[]} ("IRFs & Fit Data Map")) -> ("[Multiple Decays Fit Parameters]"=w1973:dbl[][], "[Decay Fit Parameter Names]"=w1967:T14[], "[IRFs]"=w2021:dbl[][], "IRF Array Time Axis"=w2023:dbl[], "Fit Options: Decay Preprocessing Parameters"=w1956:T15, "Fit Options: Reference Decay"=w1954:cluster{"t Array":dbl[], "I Array":dbl[]}, "[Decay Sum]"=w1924:dbl[])
                  n236 = call <vilib>:"H5Gclose.vi"("error in (no error)"=w2012, "group in"=w2013) -> ("error out"=w1989:errorcluster)  [unwired: 9 in]
                  n237 = call <vilib>:"H5Gopen.vi"("error in (no error)"=w1989, "name"="Decay Fit Options & Parameters" ("dataset name"), "ref in"=w1978) -> ("error out"=w1998:errorcluster, "group out"=w1997:T28)  [unwired: 7 in]
                  n238 = xnode "H5Dread.xnode"("dataset name (this)"="Laser Period" ("dataset name"), "error in (no error)"=w1998, "default"=w1986, "ref in"=w1997) -> ("error out"=w1940:errorcluster, "data"=w1980:dbl[unit], "ref out"=w1937:T28)  [unwired: 2 in, 1 out]
                  n239 = xnode "H5Dread.xnode"("dataset name (this)"="MLE Baseline Offset Type" ("dataset name"), "error in (no error)"=w1940, "default"=w1938, "ref in"=w1937) -> ("error out"=w1936:errorcluster, "data"=w1931:T11)  [unwired: 2 in, 2 out]
                  n240 = xnode "H5Dread.xnode"("dataset name (this)"="MLE Baseline Offset" ("dataset name"), "error in (no error)"=w1936, "default"=w1932, "ref in"=w1937) -> ("error out"=w1934:errorcluster, "data"=w1930:dbl, "ref out"=w1935:i64)  [unwired: 2 in, 1 out]
                  n241 = xnode "H5Dread.xnode"("dataset name (this)"="Fit Options" ("dataset name"), "error in (no error)"=w1934, "default"=w1985, "ref in"=w1935) -> ("error out"=w1996:errorcluster, "data"=w1981:T2, "ref out"=w1994:i64)  [unwired: 2 in, 1 out]
                  n242 = xnode "H5Dread.xnode"("dataset name (this)"="Fit Parameter Constraints" ("dataset name"), "error in (no error)"=w1996, "default"=w1984, "ref in"=w1994) -> ("error out"=w1995:errorcluster, "data"=w1982:T9[], "ref out"=w1993:T28)  [unwired: 2 in, 1 out]
                  n243 = Unbundle By Name(w1954) -> ("t Array"=w1953:dbl[], "I Array"=w1951:dbl[])
                  n244 = call <vilib>:"H5Gclose.vi"("error in (no error)"=w1995, "group in"=w1993) -> ("error out"=w1988:errorcluster)  [unwired: 9 in]
                  n245 = xnode "H5Dread.xnode"("dataset name (this)"="IRF Array Time Axis" ("dataset name"), "error in (no error)"=w1988, "default"=w2023, "ref in"=w1978) -> ("error out"=w2026:errorcluster, "data"=w2002:dbl[], "ref out"=w2025:T28)  [unwired: 2 in, 1 out]
                  n246 = xnode "H5Dread.xnode"("dataset name (this)"="IRF Array" ("dataset name"), "error in (no error)"=w2026, "default"=w2021, "ref in"=w2025) -> ("error out"=w1943:errorcluster, "data"=w2019:dbl[][], "ref out"=w2018:T28)  [unwired: 2 in, 1 out]
                  n247 = xnode "H5Dread.xnode"("dataset name (this)"=w1948, "error in (no error)"=w1943, "default"=w1967, "ref in"=w2018) -> ("error out"=w1949:errorcluster, "data"=w1946:T14[], "ref out"=w1945:T28)  [unwired: 2 in, 1 out]
                  n248 = case shown="Error .." w1949 {
                    selector: w1949 -> [w2073 _]
                    tunnel: w1945 -> [w2074 w2079]
                    tunnel: [w2074 w2083] -> w1947
                    tunnel: [w2073 w2081] -> w1944
                    tunnel: [w2072 w2077] -> w1942
                    tunnel: w1948 -> [_ w2082]
                    tunnel: w1943 -> [_ w2080]
                    tunnel: w1946 -> [w2072 _]
                    frame No Error {
                      # "New version"
                    }
                    frame Error {
                      # "version 1"
                      n249 = xnode "H5Dread.xnode"("dataset name (this)"=w2082, "error in (no error)"=w2080, "default"=u16[] [], "ref in"=w2079) -> ("error out"=w2081:errorcluster, "data"=w2076:u16[], "ref out"=w2083:i64)  [unwired: 2 in, 1 out]
                      n250 = Array Size(array=w2076) -> (size(s)=w2075:i32)
                      n251 = call "Get Valid Decay Fit Parameters List.vi"("Parameter ID Array Size"=w2075) -> ("Parameter Name Array"=w2077:T14[])
                    }
                  }
                  n252 = case shown="Error .." w1944 {
                    selector: w1944 -> [w2145 _]
                    tunnel: w1947 -> [w2146 w2155]
                    tunnel: [w2146 w2154] -> w1971
                    tunnel: [w2145 w2152] -> w1970
                    tunnel: w1942 -> [w2144 _]
                    tunnel: [w2144 w2150] -> w1969
                    tunnel: "Decay Fit Parameter Names" ("name") -> [_ w2153]
                    tunnel: w1943 -> [_ w2151]
                    frame No Error {
                      # "New version"
                    }
                    frame Error {
                      # "Old version"
                      n253 = xnode "H5Dread.xnode"("dataset name (this)"=w2153, "error in (no error)"=w2151, "default"=u16[] [], "ref in"=w2155) -> ("error out"=w2152:errorcluster, "data"=w2148:u16[], "ref out"=w2154:i64)  [unwired: 2 in, 1 out]
                      n254 = Array Size(array=w2148) -> (size(s)=w2147:i32)
                      n255 = call "Get Valid Decay Fit Parameters List.vi"("Parameter ID Array Size"=w2147) -> ("Parameter Name Array"=w2150:T14[])
                    }
                  }
                  n256 = for {
                    tunnel: w1969 -> [w2232] mode=indexing
                    tunnel: w2007 -> [w2233]
                    tunnel: [w2231] -> w2006 mode=indexing
                    n257 = Index Array(array=w2233, index=w2232) -> (element=w2231:string)
                  }
                  n258 = xnode "H5Dread.xnode"("dataset name (this)"="Multiple Decay Fit Parameters Array" ("name"), "error in (no error)"=w1970, "default"=w1973, "ref in"=w1971) -> ("error out"=w1964:errorcluster, "data"=w1974:dbl[][], "ref out"=w1965:T28)  [unwired: 2 in, 1 out]
                  n259 = xnode "H5Dread.xnode"("dataset name (this)"="Decay Preprocessing Parameters" ("name"), "error in (no error)"=w1964, "default"=w1956, "ref in"=w1965) -> ("error out"=w1961:errorcluster, "data"=w1955:T15, "ref out"=w1963:T28)  [unwired: 2 in, 1 out]
                  n260 = xnode "H5Dread.xnode"("dataset name (this)"="Reference Decay: t Array" ("name"), "error in (no error)"=w1961, "default"=w1953, "ref in"=w1963) -> ("error out"=w1960:errorcluster, "data"=w1952:dbl[], "ref out"=w1962:T28)  [unwired: 2 in, 1 out]
                  n261 = xnode "H5Dread.xnode"("dataset name (this)"="Reference Decay: I Array" ("name"), "error in (no error)"=w1960, "default"=w1951, "ref in"=w1962) -> ("error out"=w1928:errorcluster, "data"=w1950:dbl[], "ref out"=w1929:T28)  [unwired: 2 in, 1 out]
                  n262 = xnode "H5Dread.xnode"("dataset name (this)"="Decay Sums" ("name"), "error in (no error)"=w1928, "default"=w1924, "ref in"=w1929) -> ("error out"=w1926:errorcluster, "data"=w1923:dbl[], "ref out"=w1927:i64)  [unwired: 2 in, 1 out]
                  n263 = Bundle By Name(cluster=w1966, "[Multiple Decays Fit Parameters]"=w1974, "[Decay Fit Parameter Names]"=w1969, "[IRFs]"=w2019, "IRF Array Time Axis"=w2002, "Fit Options: Decay Preprocessing Parameters"=w1955, "Fit Options: Reference Decay.t Array"=w1952, "Fit Options: Reference Decay.I Array"=w1950, "[Decay Sum]"=w1923) -> (w2016:T13)
                  n264 = Array Size(array=w1974) -> (size(s)=w2001:i32[])
                  n265 = call "Concatenate String Array.vi"("Separator (TAB)"=", ", "String Array"=w2006) -> ("Formatted String"=w2004:string)  [unwired: 9 in]
                  n266 = xnode "H5Dread.xnode"("dataset name (this)"="Multiple Decay Fit Parameters SDV Array" ("name"), "error in (no error)"=w1926, "default"=w1973, "ref in"=w1927) -> ("error out"=w1977:errorcluster, "data"=w1972:dbl[][], "ref out"=w1976:T28)  [unwired: 2 in, 1 out]
                  n267 = Array Size(array=w2002) -> (size(s)=w2003:i32)
                  n268 = Index Array(array=w2001) -> (element #1=w2000:i32, element #2=w1999:i32)  [unwired: 2 in]
                  n269 = Bundle By Name(cluster=w1941, "Fit Parameter Constraints"=w1982, "Fit Options"=w1981, "SYNC Period"=w1980, "MLE Baseline Offset Type"=w1931, "MLE Baseline Offset"=w1930) -> (w1979:T1)
                  n270 = Format Into String(format string="Parameter Names: %s\nIRFs Length: %d\n# Data Points: %d x %d", initial string=w2009, error in=w1977, w2004, w2003, w2000, w1999) -> (resulting string=w2010:string, error out=w2011:errorcluster)
                }
              }
            }
            frame True {
              # "File Type & Version only"
              n271 = call <vilib>:"H5Gclose.vi"("error in (no error)"=w2297, "group in"=w2296) -> ("error out"=w2294:errorcluster)  [unwired: 9 in]
            }
          }
        }
      }
      n272 = call <vilib>:"H5Fclose.vi"("error in (no error)"=w41, "ref"=w42) -> ("error out"=w25:errorcluster)  [unwired: 9 in]
      n273 = call "High Resolution Timing.vi"("relative seconds (NaN)"=w38, "Error In"=w25) -> ("elapsed (relative) seconds"=w37:dbl, "Error Out"=w39:errorcluster)  [unwired: 15 in, 1 out]
    }
  }
  "error out" <- w13
  "elapsed (relative) seconds" <- w6
  "Data Description" <- w4
  "IRFs & Fit Data Map v3" <- w5
  "Decay Fit Options & Parameters" <- w3
  "[Multiple Decays Fit Parameters SDV]" <- w1
